vi "DIALOG_Property Selection.vi"(7 "Action":T6, 8 "Error In":errorcluster, 9 "User VI Ref":refnum<vi>, 10 "Affected Items":T4, 11 "Properties for Tree In":T5(array[cluster])=[{"Label"="Divider", "Tag"="0,6,MCListbox (strict),Divider,Divider", "Property Type"=enum."Divider", "Indent"=0, "Can Read?"=FALSE, "Can Write?"=FALSE, "Is Read?"=FALSE, "Is Write?"=FALSE, "Inactive Parent?"=FALSE, "Unwired?"=FALSE}, {"Label"="Class ID", "Tag"="1,1,MCListbox (strict),6327800,Class ID", "Property Type"=enum."Base", "Indent"=0, "Can Read?"=TRUE, "Can Write?"=FALSE, "Is Read?"=FALSE, "Is Write?"=FALSE, "Inactive Parent?"=FALSE, "Unwired?"=FALSE}, {"Label"="Class Name", "Tag"="2,1,MCListbox (strict),6327803,Class Name", "Property Type"=enum."Base", "Indent"=0, "Can Read?"=TRUE, "Can Write?"=FALSE, "Is Read?"=FALSE, "Is Write?"=FALSE, "Inactive Parent?"=FALSE, "Unwired?"=FALSE}, {"Label"="Is On Block Diagram?", "Tag"="3,2,MCListbox (strict),6327805,Is On Block Diagram?", "Property Type"=enum."Scripting", "Indent"=0, "Can Read?"=TRUE, "Can Write?"=FALSE, "Is Read?"=FALSE, "Is Write?"=FALSE, "Inactive Parent?"=FALSE, "Unwired?"=FALSE}, {"Label"="Modified", "Tag"="4,3,MCListbox (strict),6327804,Modified", "Property Type"=enum."Private", "Indent"=0, "Can Read?"=TRUE, "Can Write?"=FALSE, "Is Read?"=FALSE, "Is Write?"=FALSE, "Inactive Parent?"=FALSE, "Unwired?"=FALSE}, {"Label"="Owner", "Tag"="5,1,MCListbox (strict),6327806,Owner", "Property Type"=enum."Base", "Indent"=0, "Can Read?"=TRUE, "Can Write?"=FALSE, "Is Read?"=FALSE, "Is Write?"=FALSE, "Inactive Parent?"=FALSE, "Unwired?"=FALSE}, {"Label"="Owning VI", "Tag"="6,1,MCListbox (strict),6327802,Owning VI", "Property Type"=enum."Base", "Indent"=0, "Can Read?"=TRUE, "Can Write?"=FALSE, "Is Read?"=FALSE, "Is Write?"=FALSE, "Inactive Parent?"=FALSE, "Unwired?"=FALSE}, {"Label"="Divider", "Tag"="7,6,MCListbox (strict),Divider,Divider", "Property Type"=enum."Divider", "Indent"=0, "Can Read?"=FALSE, "Can Write?"=FALSE, "Is Read?"=FALSE, "Is Write?"=FALSE, "Inactive Parent?"=FALSE, "Unwired?"=FALSE}, {"Label"="Basic Object Flags", "Tag"="8,3,MCListbox (strict),632a80c,Basic Object Flags", "Property Type"=enum."Private", "Indent"=0, "Can Read?"=TRUE, "Can Write?"=TRUE, "Is Read?"=FALSE, "Is Write?"=FALSE, "Inactive Parent?"=FALSE, "Unwired?"=FALSE}, {"Label"="Bounds", "Tag"="9,1,MCListbox (strict),632a803,Bounds", "Property Type"=enum."Base", "Indent"=0, "Can Read?"=TRUE, "Can Write?"=FALSE, "Is Read?"=FALSE, "Is Write?"=FALSE, "Inactive Parent?"=FALSE, "Unwired?"=FALSE}, {"Label"="Area Height", "Tag"="10,1,MCListbox (strict),632a805,Bounds:Area Height", "Property Type"=enum."Base", "Indent"=1, "Can Read?"=TRUE, "Can Write?"=FALSE, "Is Read?"=FALSE, "Is Write?"=FALSE, "Inactive Parent?"=FALSE, "Unwired?"=FALSE}, {"Label"="Area Width", "Tag"="11,1,MCListbox (strict),632a804,Bounds:Area Width", "Property Type"=enum."Base", "Indent"=1, "Can Read?"=TRUE, "Can Write?"=FALSE, "Is Read?"=FALSE, "Is Write?"=FALSE, "Inactive Parent?"=FALSE, "Unwired?"=FALSE}, {"Label"="Dependencies", "Tag"="12,2,MCListbox (strict),632a817,Dependencies", "Property Type"=enum."None", "Indent"=0, "Can Read?"=FALSE, "Can Write?"=FALSE, "Is Read?"=FALSE, "Is Write?"=FALSE, "Inactive Parent?"=TRUE, "Unwired?"=FALSE}, {"Label"="Found Dependency Names", "Tag"="13,2,MCListbox (strict),632a817,Dependencies:Found Dependency Names", "Property Type"=enum."Scripting", "Indent"=1, "Can Read?"=TRUE, "Can Write?"=FALSE, "Is Read?"=FALSE, "Is Write?"=FALSE, "Inactive Parent?"=FALSE, "Unwired?"=FALSE}, {"Label"="Found Dependency Paths", "Tag"="14,2,MCListbox (strict),632a816,Dependencies:Found Dependency Paths", "Property Type"=enum."Scripting", "Indent"=1, "Can Read?"=TRUE, "Can Write?"=FALSE, "Is Read?"=FALSE, "Is Write?"=FALSE, "Inactive Parent?"=FALSE, "Unwired?"=FALSE}, {"Label"="Missing Dependency Names", "Tag"="15,2,MCListbox (strict),632a815,Dependencies:Missing Dependency Names", "Property Type"=enum."Scripting", "Indent"=1, "Can Read?"=TRUE, "Can Write?"=FALSE, "Is Read?"=FALSE, "Is Write?"=FALSE, "Inactive Parent?"=FALSE, "Unwired?"=FALSE}, {"Label"="Missing Dependency Paths", "Tag"="16,2,MCListbox (strict),632a814,Dependencies:Missing Dependency Paths", "Property Type"=enum."Scripting", "Indent"=1, "Can Read?"=TRUE, "Can Write?"=FALSE, "Is Read?"=FALSE, "Is Write?"=FALSE, "Inactive Parent?"=FALSE, "Unwired?"=FALSE}, {"Label"="Group Member Refs[]", "Tag"="17,3,MCListbox (strict),632a808,Group Member Refs[]", "Property Type"=enum."Private", "Indent"=0, "Can Read?"=TRUE, "Can Write?"=FALSE, "Is Read?"=FALSE, "Is Write?"=FALSE, "Inactive Parent?"=FALSE, "Unwired?"=FALSE}, {"Label"="Grouped", "Tag"="18,3,MCListbox (strict),632a806,Grouped", "Property Type"=enum."Private", "Indent"=0, "Can Read?"=TRUE, "Can Write?"=FALSE, "Is Read?"=FALSE, "Is Write?"=FALSE, "Inactive Parent?"=FALSE, "Unwired?"=FALSE}, {"Label"="Is Wizard Locked", "Tag"="19,3,MCListbox (strict),632a80d,Is Wizard Locked", "Property Type"=enum."Private", "Indent"=0, "Can Read?"=TRUE, "Can Write?"=FALSE, "Is Read?"=FALSE, "Is Write?"=FALSE, "Inactive Parent?"=FALSE, "Unwired?"=FALSE}, {"Label"="Locked", "Tag"="20,3,MCListbox (strict),632a807,Locked", "Property Type"=enum."Private", "Indent"=0, "Can Read?"=TRUE, "Can Write?"=FALSE, "Is Read?"=FALSE, "Is Write?"=FALSE, "Inactive Parent?"=FALSE, "Unwired?"=FALSE}, {"Label"="Master Bounds Rect", "Tag"="21,2,MCListbox (strict),632a80b,Master Bounds Rect", "Property Type"=enum."Scripting", "Indent"=0, "Can Read?"=TRUE, "Can Write?"=FALSE, "Is Read?"=FALSE, "Is Write?"=FALSE, "Inactive Parent?"=FALSE, "Unwired?"=FALSE}, {"Label"="Position", "Tag"="22,1,MCListbox (strict),632a800,Position", "Property Type"=enum."Base", "Indent"=0, "Can Read?"=TRUE, "Can Write?"=TRUE, "Is Read?"=FALSE, "Is Write?"=FALSE, "Inactive Parent?"=FALSE, "Unwired?"=FALSE}, {"Label"="Left", "Tag"="23,1,MCListbox (strict),632a801,Position:Left", "Property Type"=enum."Base", "Indent"=1, "Can Read?"=TRUE, "Can Write?"=TRUE, "Is Read?"=FALSE, "Is Write?"=FALSE, "Inactive Parent?"=FALSE, "Unwired?"=FALSE}, {"Label"="Top", "Tag"="24,1,MCListbox (strict),632a802,Position:Top", "Property Type"=enum."Base", "Indent"=1, "Can Read?"=TRUE, "Can Write?"=TRUE, "Is Read?"=FALSE, "Is Write?"=FALSE, "Inactive Parent?"=FALSE, "Unwired?"=FALSE}, {"Label"="Resize Info", "Tag"="25,3,MCListbox (strict),632a80f,Resize Info", "Property Type"=enum."None", "Indent"=0, "Can Read?"=FALSE, "Can Write?"=FALSE, "Is Read?"=FALSE, "Is Write?"=FALSE, "Inactive Parent?"=TRUE, "Unwired?"=FALSE}, {"Label"="Can Resize Horizontally", "Tag"="26,3,MCListbox (strict),632a80f,Resize Info:Can Resize Horizontally", "Property Type"=enum."Private", "Indent"=1, "Can Read?"=TRUE, "Can Write?"=FALSE, "Is Read?"=FALSE, "Is Write?"=FALSE, "Inactive Parent?"=FALSE, "Unwired?"=FALSE}, {"Label"="Can Resize Vertically", "Tag"="27,3,MCListbox (strict),632a810,Resize Info:Can Resize Vertically", "Property Type"=enum."Private", "Indent"=1, "Can Read?"=TRUE, "Can Write?"=FALSE, "Is Read?"=FALSE, "Is Write?"=FALSE, "Inactive Parent?"=FALSE, "Unwired?"=FALSE}, {"Label"="Include In Resize", "Tag"="28,3,MCListbox (strict),632a812,Resize Info:Include In Resize", "Property Type"=enum."Private", "Indent"=1, "Can Read?"=TRUE, "Can Write?"=FALSE, "Is Read?"=FALSE, "Is Write?"=FALSE, "Inactive Parent?"=FALSE, "Unwired?"=FALSE}, {"Label"="Name in Resize Dialog", "Tag"="29,3,MCListbox (strict),632a811,Resize Info:Name in Resize Dialog", "Property Type"=enum."Private", "Indent"=1, "Can Read?"=TRUE, "Can Write?"=FALSE, "Is Read?"=FALSE, "Is Write?"=FALSE, "Inactive Parent?"=FALSE, "Unwired?"=FALSE}, {"Label"="Selected", "Tag"="30,2,MCListbox (strict),632a809,Selected", "Property Type"=enum."Scripting", "Indent"=0, "Can Read?"=TRUE, "Can Write?"=TRUE, "Is Read?"=FALSE, "Is Write?"=FALSE, "Inactive Parent?"=FALSE, "Unwired?"=FALSE}, {"Label"="Total Bounds Rect", "Tag"="31,2,MCListbox (strict),632a80a,Total Bounds Rect", "Property Type"=enum."Scripting", "Indent"=0, "Can Read?"=TRUE, "Can Write?"=FALSE, "Is Read?"=FALSE, "Is Write?"=FALSE, "Inactive Parent?"=FALSE, "Unwired?"=FALSE}, {"Label"="UID", "Tag"="32,2,MCListbox (strict),632a813,UID", "Property Type"=enum."Scripting", "Indent"=0, "Can Read?"=TRUE, "Can Write?"=FALSE, "Is Read?"=FALSE, "Is Write?"=FALSE, "Inactive Parent?"=FALSE, "Unwired?"=FALSE}, {"Label"="Divider", "Tag"="33,6,MCListbox (strict),Divider,Divider", "Property Type"=enum."Divider", "Indent"=0, "Can Read?"=FALSE, "Can Write?"=FALSE, "Is Read?"=FALSE, "Is Write?"=FALSE, "Inactive Parent?"=FALSE, "Unwired?"=FALSE}, {"Label"="Auto-Update From Typedef", "Tag"="34,2,MCListbox (strict),633201c,Auto-Update From Typedef", "Property Type"=enum."Scripting", "Indent"=0, "Can Read?"=TRUE, "Can Write?"=TRUE, "Is Read?"=FALSE, "Is Write?"=FALSE, "Inactive Parent?"=FALSE, "Unwired?"=FALSE}, {"Label"="Bit Accurate Data Size", "Tag"="35,3,MCListbox (strict),633201d,Bit Accurate Data Size", "Property Type"=enum."Private", "Indent"=0, "Can Read?"=TRUE, "Can Write?"=FALSE, "Is Read?"=FALSE, "Is Write?"=FALSE, "Inactive Parent?"=FALSE, "Unwired?"=FALSE}, {"Label"="Blinking", "Tag"="36,1,MCListbox (strict),6332003,Blinking", "Property Type"=enum."Base", "Indent"=0, "Can Read?"=TRUE, "Can Write?"=TRUE, "Is Read?"=FALSE, "Is Write?"=FALSE, "Inactive Parent?"=FALSE, "Unwired?"=FALSE}, {"Label"="Built-In Mouse Wheel Support", "Tag"="37,1,MCListbox (strict),633203f,Built-In Mouse Wheel Support", "Property Type"=enum."Base", "Indent"=0, "Can Read?"=TRUE, "Can Write?"=TRUE, "Is Read?"=FALSE, "Is Write?"=FALSE, "Inactive Parent?"=FALSE, "Unwired?"=FALSE}, {"Label"="C Type", "Tag"="38,3,MCListbox (strict),6332026,C Type", "Property Type"=enum."Private", "Indent"=0, "Can Read?"=TRUE, "Can Write?"=FALSE, "Is Read?"=FALSE, "Is Write?"=FALSE, "Inactive Parent?"=FALSE, "Unwired?"=FALSE}, {"Label"="Caption", "Tag"="39,1,MCListbox (strict),6332004,Caption", "Property Type"=enum."Base", "Indent"=0, "Can Read?"=TRUE, "Can Write?"=FALSE, "Is Read?"=FALSE, "Is Write?"=FALSE, "Inactive Parent?"=FALSE, "Unwired?"=FALSE}, {"Label"="Class ID", "Tag"="40,1,MCListbox (strict),6332004.6327800,Caption.Class ID", "Property Type"=enum."Base", "Indent"=1, "Can Read?"=TRUE, "Can Write?"=FALSE, "Is Read?"=FALSE, "Is Write?"=FALSE, "Inactive Parent?"=FALSE, "Unwired?"=FALSE}, {"Label"="Class Name", "Tag"="41,1,MCListbox (strict),6332004.6327803,Caption.Class Name", "Property Type"=enum."Base", "Indent"=1, "Can Read?"=TRUE, "Can Write?"=FALSE, "Is Read?"=FALSE, "Is Write?"=FALSE, "Inactive Parent?"=FALSE, "Unwired?"=FALSE}, {"Label"="Is On Block Diagram?", "Tag"="42,2,MCListbox (strict),6332004.6327805,Caption.Is On Block Diagram?", "Property Type"=enum."Scripting", "Indent"=1, "Can Read?"=TRUE, "Can Write?"=FALSE, "Is Read?"=FALSE, "Is Write?"=FALSE, "Inactive Parent?"=FALSE, "Unwired?"=FALSE}, {"Label"="Modified", "Tag"="43,3,MCListbox (strict),6332004.6327804,Caption.Modified", "Property Type"=enum."Private", "Indent"=1, "Can Read?"=TRUE, "Can Write?"=FALSE, "Is Read?"=FALSE, "Is Write?"=FALSE, "Inactive Parent?"=FALSE, "Unwired?"=FALSE}, {"Label"="Owner", "Tag"="44,1,MCListbox (strict),6332004.6327806,Caption.Owner", "Property Type"=enum."Base", "Indent"=1, "Can Read?"=TRUE, "Can Write?"=FALSE, "Is Read?"=FALSE, "Is Write?"=FALSE, "Inactive Parent?"=FALSE, "Unwired?"=FALSE}, {"Label"="Owning VI", "Tag"="45,1,MCListbox (strict),6332004.6327802,Caption.Owning VI", "Property Type"=enum."Base", "Indent"=1, "Can Read?"=TRUE, "Can Write?"=FALSE, "Is Read?"=FALSE, "Is Write?"=FALSE, "Inactive Parent?"=FALSE, "Unwired?"=FALSE}, {"Label"="Basic Object Flags", "Tag"="46,3,MCListbox (strict),6332004.632a80c,Caption.Basic Object Flags", "Property Type"=enum."Private", "Indent"=1, "Can Read?"=TRUE, "Can Write?"=TRUE, "Is Read?"=FALSE, "Is Write?"=FALSE, "Inactive Parent?"=FALSE, "Unwired?"=FALSE}, {"Label"="Bounds", "Tag"="47,1,MCListbox (strict),6332004.632a803,Caption.Bounds", "Property Type"=enum."Base", "Indent"=1, "Can Read?"=TRUE, "Can Write?"=FALSE, "Is Read?"=FALSE, "Is Write?"=FALSE, "Inactive Parent?"=FALSE, "Unwired?"=FALSE}, {"Label"="Area Height", "Tag"="48,1,MCListbox (strict),6332004.632a805,Caption.Bounds:Area Height", "Property Type"=enum."Base", "Indent"=2, "Can Read?"=TRUE, "Can Write?"=FALSE, "Is Read?"=FALSE, "Is Write?"=FALSE, "Inactive Parent?"=FALSE, "Unwired?"=FALSE}, {"Label"="Area Width", "Tag"="49,1,MCListbox (strict),6332004.632a804,Caption.Bounds:Area Width", "Property Type"=enum."Base", "Indent"=2, "Can Read?"=TRUE, "Can Write?"=FALSE, "Is Read?"=FALSE, "Is Write?"=FALSE, "Inactive Parent?"=FALSE, "Unwired?"=FALSE}, {"Label"="Dependencies", "Tag"="50,2,MCListbox (strict),6332004.632a817,Caption.Dependencies", "Property Type"=enum."None", "Indent"=1, "Can Read?"=FALSE, "Can Write?"=FALSE, "Is Read?"=FALSE, "Is Write?"=FALSE, "Inactive Parent?"=TRUE, "Unwired?"=FALSE}, {"Label"="Found Dependency Names", "Tag"="51,2,MCListbox (strict),6332004.632a817,Caption.Dependencies:Found Dependency Names", "Property Type"=enum."Scripting", "Indent"=2, "Can Read?"=TRUE, "Can Write?"=FALSE, "Is Read?"=FALSE, "Is Write?"=FALSE, "Inactive Parent?"=FALSE, "Unwired?"=FALSE}, {"Label"="Found Dependency Paths", "Tag"="52,2,MCListbox (strict),6332004.632a816,Caption.Dependencies:Found Dependency Paths", "Property Type"=enum."Scripting", "Indent"=2, "Can Read?"=TRUE, "Can Write?"=FALSE, "Is Read?"=FALSE, "Is Write?"=FALSE, "Inactive Parent?"=FALSE, "Unwired?"=FALSE}, {"Label"="Missing Dependency Names", "Tag"="53,2,MCListbox (strict),6332004.632a815,Caption.Dependencies:Missing Dependency Names", "Property Type"=enum."Scripting", "Indent"=2, "Can Read?"=TRUE, "Can Write?"=FALSE, "Is Read?"=FALSE, "Is Write?"=FALSE, "Inactive Parent?"=FALSE, "Unwired?"=FALSE}, {"Label"="Missing Dependency Paths", "Tag"="54,2,MCListbox (strict),6332004.632a814,Caption.Dependencies:Missing Dependency Paths", "Property Type"=enum."Scripting", "Indent"=2, "Can Read?"=TRUE, "Can Write?"=FALSE, "Is Read?"=FALSE, "Is Write?"=FALSE, "Inactive Parent?"=FALSE, "Unwired?"=FALSE}, {"Label"="Group Member Refs[]", "Tag"="55,3,MCListbox (strict),6332004.632a808,Caption.Group Member Refs[]", "Property Type"=enum."Private", "Indent"=1, "Can Read?"=TRUE, "Can Write?"=FALSE, "Is Read?"=FALSE, "Is Write?"=FALSE, "Inactive Parent?"=FALSE, "Unwired?"=FALSE}, {"Label"="Grouped", "Tag"="56,3,MCListbox (strict),6332004.632a806,Caption.Grouped", "Property Type"=enum."Private", "Indent"=1, "Can Read?"=TRUE, "Can Write?"=FALSE, "Is Read?"=FALSE, "Is Write?"=FALSE, "Inactive Parent?"=FALSE, "Unwired?"=FALSE}, {"Label"="Is Wizard Locked", "Tag"="57,3,MCListbox (strict),6332004.632a80d,Caption.Is Wizard Locked", "Property Type"=enum."Private", "Indent"=1, "Can Read?"=TRUE, "Can Write?"=FALSE, "Is Read?"=FALSE, "Is Write?"=FALSE, "Inactive Parent?"=FALSE, "Unwired?"=FALSE}, {"Label"="Locked", "Tag"="58,3,MCListbox (strict),6332004.632a807,Caption.Locked", "Property Type"=enum."Private", "Indent"=1, "Can Read?"=TRUE, "Can Write?"=FALSE, "Is Read?"=FALSE, "Is Write?"=FALSE, "Inactive Parent?"=FALSE, "Unwired?"=FALSE}, {"Label"="Master Bounds Rect", "Tag"="59,2,MCListbox (strict),6332004.632a80b,Caption.Master Bounds Rect", "Property Type"=enum."Scripting", "Indent"=1, "Can Read?"=TRUE, "Can Write?"=FALSE, "Is Read?"=FALSE, "Is Write?"=FALSE, "Inactive Parent?"=FALSE, "Unwired?"=FALSE}, {"Label"="Position", "Tag"="60,1,MCListbox (strict),6332004.632a800,Caption.Position", "Property Type"=enum."Base", "Indent"=1, "Can Read?"=TRUE, "Can Write?"=TRUE, "Is Read?"=FALSE, "Is Write?"=FALSE, "Inactive Parent?"=FALSE, "Unwired?"=FALSE}, {"Label"="Left", "Tag"="61,1,MCListbox (strict),6332004.632a801,Caption.Position:Left", "Property Type"=enum."Base", "Indent"=2, "Can Read?"=TRUE, "Can Write?"=TRUE, "Is Read?"=FALSE, "Is Write?"=FALSE, "Inactive Parent?"=FALSE, "Unwired?"=FALSE}, {"Label"="Top", "Tag"="62,1,MCListbox (strict),6332004.632a802,Caption.Position:Top", "Property Type"=enum."Base", "Indent"=2, "Can Read?"=TRUE, "Can Write?"=TRUE, "Is Read?"=FALSE, "Is Write?"=FALSE, "Inactive Parent?"=FALSE, "Unwired?"=FALSE}, {"Label"="Resize Info", "Tag"="63,3,MCListbox (strict),6332004.632a80f,Caption.Resize Info", "Property Type"=enum."None", "Indent"=1, "Can Read?"=FALSE, "Can Write?"=FALSE, "Is Read?"=FALSE, "Is Write?"=FALSE, "Inactive Parent?"=TRUE, "Unwired?"=FALSE}, {"Label"="Can Resize Horizontally", "Tag"="64,3,MCListbox (strict),6332004.632a80f,Caption.Resize Info:Can Resize Horizontally", "Property Type"=enum."Private", "Indent"=2, "Can Read?"=TRUE, "Can Write?"=FALSE, "Is Read?"=FALSE, "Is Write?"=FALSE, "Inactive Parent?"=FALSE, "Unwired?"=FALSE}, {"Label"="Can Resize Vertically", "Tag"="65,3,MCListbox (strict),6332004.632a810,Caption.Resize Info:Can Resize Vertically", "Property Type"=enum."Private", "Indent"=2, "Can Read?"=TRUE, "Can Write?"=FALSE, "Is Read?"=FALSE, "Is Write?"=FALSE, "Inactive Parent?"=FALSE, "Unwired?"=FALSE}, {"Label"="Include In Resize", "Tag"="66,3,MCListbox (strict),6332004.632a812,Caption.Resize Info:Include In Resize", "Property Type"=enum."Private", "Indent"=2, "Can Read?"=TRUE, "Can Write?"=FALSE, "Is Read?"=FALSE, "Is Write?"=FALSE, "Inactive Parent?"=FALSE, "Unwired?"=FALSE}, {"Label"="Name in Resize Dialog", "Tag"="67,3,MCListbox (strict),6332004.632a811,Caption.Resize Info:Name in Resize Dialog", "Property Type"=enum."Private", "Indent"=2, "Can Read?"=TRUE, "Can Write?"=FALSE, "Is Read?"=FALSE, "Is Write?"=FALSE, "Inactive Parent?"=FALSE, "Unwired?"=FALSE}, {"Label"="Selected", "Tag"="68,2,MCListbox (strict),6332004.632a809,Caption.Selected", "Property Type"=enum."Scripting", "Indent"=1, "Can Read?"=TRUE, "Can Write?"=TRUE, "Is Read?"=FALSE, "Is Write?"=FALSE, "Inactive Parent?"=FALSE, "Unwired?"=FALSE}, {"Label"="Total Bounds Rect", "Tag"="69,2,MCListbox (strict),6332004.632a80a,Caption.Total Bounds Rect", "Property Type"=enum."Scripting", "Indent"=1, "Can Read?"=TRUE, "Can Write?"=FALSE, "Is Read?"=FALSE, "Is Write?"=FALSE, "Inactive Parent?"=FALSE, "Unwired?"=FALSE}, {"Label"="UID", "Tag"="70,2,MCListbox (strict),6332004.632a813,Caption.UID", "Property Type"=enum."Scripting", "Indent"=1, "Can Read?"=TRUE, "Can Write?"=FALSE, "Is Read?"=FALSE, "Is Write?"=FALSE, "Inactive Parent?"=FALSE, "Unwired?"=FALSE}, {"Label"="Colors", "Tag"="71,1,MCListbox (strict),6332004.632cc03,Caption.Colors", "Property Type"=enum."Base", "Indent"=1, "Can Read?"=TRUE, "Can Write?"=TRUE, "Is Read?"=FALSE, "Is Write?"=FALSE, "Inactive Parent?"=FALSE, "Unwired?"=FALSE}, {"Label"="BG Color", "Tag"="72,1,MCListbox (strict),6332004.632cc05,Caption.Colors:BG Color", "Property Type"=enum."Base", "Indent"=2, "Can Read?"=TRUE, "Can Write?"=TRUE, "Is Read?"=FALSE, "Is Write?"=FALSE, "Inactive Parent?"=FALSE, "Unwired?"=FALSE}, {"Label"="FG Color", "Tag"="73,1,MCListbox (strict),6332004.632cc04,Caption.Colors:FG Color", "Property Type"=enum."Base", "Indent"=2, "Can Read?"=TRUE, "Can Write?"=TRUE, "Is Read?"=FALSE, "Is Write?"=FALSE, "Inactive Parent?"=FALSE, "Unwired?"=FALSE}, {"Label"="Owning Pane", "Tag"="74,1,MCListbox (strict),6332004.632cc07,Caption.Owning Pane", "Property Type"=enum."Base", "Indent"=1, "Can Read?"=TRUE, "Can Write?"=FALSE, "Is Read?"=FALSE, "Is Write?"=FALSE, "Inactive Parent?"=FALSE, "Unwired?"=FALSE}, {"Label"="Size", "Tag"="75,1,MCListbox (strict),6332004.632cc00,Caption.Size", "Property Type"=enum."Base", "Indent"=1, "Can Read?"=TRUE, "Can Write?"=TRUE, "Is Read?"=FALSE, "Is Write?"=FALSE, "Inactive Parent?"=FALSE, "Unwired?"=FALSE}, {"Label"="Height", "Tag"="76,1,MCListbox (strict),6332004.632cc02,Caption.Size:Height", "Property Type"=enum."Base", "Indent"=2, "Can Read?"=TRUE, "Can Write?"=TRUE, "Is Read?"=FALSE, "Is Write?"=FALSE, "Inactive Parent?"=FALSE, "Unwired?"=FALSE}, {"Label"="Width", "Tag"="77,1,MCListbox (strict),6332004.632cc01,Caption.Size:Width", "Property Type"=enum."Base", "Indent"=2, "Can Read?"=TRUE, "Can Write?"=TRUE, "Is Read?"=FALSE, "Is Write?"=FALSE, "Inactive Parent?"=FALSE, "Unwired?"=FALSE}, {"Label"="Visible", "Tag"="78,1,MCListbox (strict),6332004.632cc06,Caption.Visible", "Property Type"=enum."Base", "Indent"=1, "Can Read?"=TRUE, "Can Write?"=TRUE, "Is Read?"=FALSE, "Is Write?"=FALSE, "Inactive Parent?"=FALSE, "Unwired?"=FALSE}, {"Label"="Attached Object", "Tag"="79,1,MCListbox (strict),6332004.632d819,Caption.Attached Object", "Property Type"=enum."Base", "Indent"=1, "Can Read?"=TRUE, "Can Write?"=TRUE, "Is Read?"=FALSE, "Is Write?"=FALSE, "Inactive Parent?"=FALSE, "Unwired?"=FALSE}, {"Label"="Document Bounds", "Tag"="80,2,MCListbox (strict),6332004.632d812,Caption.Document Bounds", "Property Type"=enum."Scripting", "Indent"=1, "Can Read?"=TRUE, "Can Write?"=FALSE, "Is Read?"=FALSE, "Is Write?"=FALSE, "Inactive Parent?"=FALSE, "Unwired?"=FALSE}, {"Label"="Height", "Tag"="81,2,MCListbox (strict),6332004.632d814,Caption.Document Bounds:Height", "Property Type"=enum."Scripting", "Indent"=2, "Can Read?"=TRUE, "Can Write?"=FALSE, "Is Read?"=FALSE, "Is Write?"=FALSE, "Inactive Parent?"=FALSE, "Unwired?"=FALSE}, {"Label"="Width", "Tag"="82,2,MCListbox (strict),6332004.632d813,Caption.Document Bounds:Width", "Property Type"=enum."Scripting", "Indent"=2, "Can Read?"=TRUE, "Can Write?"=FALSE, "Is Read?"=FALSE, "Is Write?"=FALSE, "Inactive Parent?"=FALSE, "Unwired?"=FALSE}, {"Label"="Enable Hyperlinks", "Tag"="83,1,MCListbox (strict),6332004.632d81a,Caption.Enable Hyperlinks", "Property Type"=enum."Base", "Indent"=1, "Can Read?"=TRUE, "Can Write?"=TRUE, "Is Read?"=FALSE, "Is Write?"=FALSE, "Inactive Parent?"=FALSE, "Unwired?"=FALSE}, {"Label"="Font", "Tag"="84,1,MCListbox (strict),6332004.632d801,Caption.Font", "Property Type"=enum."Base", "Indent"=1, "Can Read?"=TRUE, "Can Write?"=TRUE, "Is Read?"=FALSE, "Is Write?"=FALSE, "Inactive Parent?"=FALSE, "Unwired?"=FALSE}, {"Label"="Bold", "Tag"="85,1,MCListbox (strict),6332004.632d809,Caption.Font:Bold", "Property Type"=enum."Base", "Indent"=2, "Can Read?"=TRUE, "Can Write?"=TRUE, "Is Read?"=FALSE, "Is Write?"=FALSE, "Inactive Parent?"=FALSE, "Unwired?"=FALSE}, {"Label"="Color", "Tag"="86,1,MCListbox (strict),6332004.632d80d,Caption.Font:Color", "Property Type"=enum."Base", "Indent"=2, "Can Read?"=TRUE, "Can Write?"=TRUE, "Is Read?"=FALSE, "Is Write?"=FALSE, "Inactive Parent?"=FALSE, "Unwired?"=FALSE}, {"Label"="Italic", "Tag"="87,1,MCListbox (strict),6332004.632d80a,Caption.Font:Italic", "Property Type"=enum."Base", "Indent"=2, "Can Read?"=TRUE, "Can Write?"=TRUE, "Is Read?"=FALSE, "Is Write?"=FALSE, "Inactive Parent?"=FALSE, "Unwired?"=FALSE}, {"Label"="Name", "Tag"="88,1,MCListbox (strict),6332004.632d807,Caption.Font:Name", "Property Type"=enum."Base", "Indent"=2, "Can Read?"=TRUE, "Can Write?"=TRUE, "Is Read?"=FALSE, "Is Write?"=FALSE, "Inactive Parent?"=FALSE, "Unwired?"=FALSE}, {"Label"="Size", "Tag"="89,1,MCListbox (strict),6332004.632d808,Caption.Font:Size", "Property Type"=enum."Base", "Indent"=2, "Can Read?"=TRUE, "Can Write?"=TRUE, "Is Read?"=FALSE, "Is Write?"=FALSE, "Inactive Parent?"=FALSE, "Unwired?"=FALSE}, {"Label"="Strikeout", "Tag"="90,1,MCListbox (strict),6332004.632d80c,Caption.Font:Strikeout", "Property Type"=enum."Base", "Indent"=2, "Can Read?"=TRUE, "Can Write?"=TRUE, "Is Read?"=FALSE, "Is Write?"=FALSE, "Inactive Parent?"=FALSE, "Unwired?"=FALSE}, {"Label"="Underline", "Tag"="91,1,MCListbox (strict),6332004.632d80b,Caption.Font:Underline", "Property Type"=enum."Base", "Indent"=2, "Can Read?"=TRUE, "Can Write?"=TRUE, "Is Read?"=FALSE, "Is Write?"=FALSE, "Inactive Parent?"=FALSE, "Unwired?"=FALSE}, {"Label"="FontType", "Tag"="92,3,MCListbox (strict),6332004.632d818,Caption.FontType", "Property Type"=enum."Private", "Indent"=1, "Can Read?"=FALSE, "Can Write?"=TRUE, "Is Read?"=FALSE, "Is Write?"=FALSE, "Inactive Parent?"=FALSE, "Unwired?"=FALSE}, {"Label"="Interpret As Unicode", "Tag"="93,3,MCListbox (strict),6332004.632d811,Caption.Interpret As Unicode", "Property Type"=enum."Private", "Indent"=1, "Can Read?"=TRUE, "Can Write?"=TRUE, "Is Read?"=FALSE, "Is Write?"=FALSE, "Inactive Parent?"=FALSE, "Unwired?"=FALSE}, {"Label"="Justification", "Tag"="94,1,MCListbox (strict),6332004.632d815,Caption.Justification", "Property Type"=enum."Base", "Indent"=1, "Can Read?"=TRUE, "Can Write?"=TRUE, "Is Read?"=FALSE, "Is Write?"=FALSE, "Inactive Parent?"=FALSE, "Unwired?"=FALSE}, {"Label"="Lock", "Tag"="95,1,MCListbox (strict),6332004.632d817,Caption.Lock", "Property Type"=enum."Base", "Indent"=1, "Can Read?"=TRUE, "Can Write?"=TRUE, "Is Read?"=FALSE, "Is Write?"=FALSE, "Inactive Parent?"=FALSE, "Unwired?"=FALSE}, {"Label"="Scroll Position", "Tag"="96,1,MCListbox (strict),6332004.632d805,Caption.Scroll Position", "Property Type"=enum."Base", "Indent"=1, "Can Read?"=TRUE, "Can Write?"=TRUE, "Is Read?"=FALSE, "Is Write?"=FALSE, "Inactive Parent?"=FALSE, "Unwired?"=FALSE}, {"Label"="Selection", "Tag"="97,1,MCListbox (strict),6332004.632d802,Caption.Selection", "Property Type"=enum."Base", "Indent"=1, "Can Read?"=TRUE, "Can Write?"=TRUE, "Is Read?"=FALSE, "Is Write?"=FALSE, "Inactive Parent?"=FALSE, "Unwired?"=FALSE}, {"Label"="End", "Tag"="98,1,MCListbox (strict),6332004.632d804,Caption.Selection:End", "Property Type"=enum."Base", "Indent"=2, "Can Read?"=TRUE, "Can Write?"=TRUE, "Is Read?"=FALSE, "Is Write?"=FALSE, "Inactive Parent?"=FALSE, "Unwired?"=FALSE}, {"Label"="Start", "Tag"="99,1,MCListbox (strict),6332004.632d803,Caption.Selection:Start", "Property Type"=enum."Base", "Indent"=2, "Can Read?"=TRUE, "Can Write?"=TRUE, "Is Read?"=FALSE, "Is Write?"=FALSE, "Inactive Parent?"=FALSE, "Unwired?"=FALSE}, {"Label"="Size to Text?", "Tag"="100,1,MCListbox (strict),6332004.632d806,Caption.Size to Text?", "Property Type"=enum."Base", "Indent"=1, "Can Read?"=TRUE, "Can Write?"=TRUE, "Is Read?"=FALSE, "Is Write?"=FALSE, "Inactive Parent?"=FALSE, "Unwired?"=FALSE}, {"Label"="Text", "Tag"="101,1,MCListbox (strict),6332004.632d800,Caption.Text", "Property Type"=enum."Base", "Indent"=1, "Can Read?"=TRUE, "Can Write?"=TRUE, "Is Read?"=FALSE, "Is Write?"=FALSE, "Inactive Parent?"=FALSE, "Unwired?"=FALSE}, {"Label"="Text Colors", "Tag"="102,1,MCListbox (strict),6332004.632d80e,Caption.Text Colors", "Property Type"=enum."Base", "Indent"=1, "Can Read?"=TRUE, "Can Write?"=TRUE, "Is Read?"=FALSE, "Is Write?"=FALSE, "Inactive Parent?"=FALSE, "Unwired?"=FALSE}, {"Label"="BG Color", "Tag"="103,1,MCListbox (strict),6332004.632d810,Caption.Text Colors:BG Color", "Property Type"=enum."Base", "Indent"=2, "Can Read?"=TRUE, "Can Write?"=TRUE, "Is Read?"=FALSE, "Is Write?"=FALSE, "Inactive Parent?"=FALSE, "Unwired?"=FALSE}, {"Label"="Text Color", "Tag"="104,1,MCListbox (strict),6332004.632d80f,Caption.Text Colors:Text Color", "Property Type"=enum."Base", "Indent"=2, "Can Read?"=TRUE, "Can Write?"=TRUE, "Is Read?"=FALSE, "Is Write?"=FALSE, "Inactive Parent?"=FALSE, "Unwired?"=FALSE}, {"Label"="Text Overflow", "Tag"="105,1,MCListbox (strict),6332004.632d81b,Caption.Text Overflow", "Property Type"=enum."Base", "Indent"=1, "Can Read?"=TRUE, "Can Write?"=TRUE, "Is Read?"=FALSE, "Is Write?"=FALSE, "Inactive Parent?"=FALSE, "Unwired?"=FALSE}, {"Label"="Vertical Arrangement", "Tag"="106,1,MCListbox (strict),6332004.632d816,Caption.Vertical Arrangement", "Property Type"=enum."Base", "Indent"=1, "Can Read?"=TRUE, "Can Write?"=TRUE, "Is Read?"=FALSE, "Is Write?"=FALSE, "Inactive Parent?"=FALSE, "Unwired?"=FALSE}, {"Label"="Control Index", "Tag"="107,1,MCListbox (strict),6332040,Control Index", "Property Type"=enum."Base", "Indent"=0, "Can Read?"=TRUE, "Can Write?"=FALSE, "Is Read?"=FALSE, "Is Write?"=FALSE, "Inactive Parent?"=FALSE, "Unwired?"=FALSE}, {"Label"="Control Reference Nodes[]", "Tag"="108,2,MCListbox (strict),6332009,Control Reference Nodes[]", "Property Type"=enum."Scripting", "Indent"=0, "Can Read?"=TRUE, "Can Write?"=FALSE, "Is Read?"=FALSE, "Is Write?"=FALSE, "Inactive Parent?"=FALSE, "Unwired?"=FALSE}, {"Label"="Data Binding", "Tag"="109,1,MCListbox (strict),633202d,Data Binding", "Property Type"=enum."None", "Indent"=0, "Can Read?"=FALSE, "Can Write?"=FALSE, "Is Read?"=FALSE, "Is Write?"=FALSE, "Inactive Parent?"=TRUE, "Unwired?"=FALSE}, {"Label"="Binding Type", "Tag"="110,1,MCListbox (strict),633202d,Data Binding:Binding Type", "Property Type"=enum."Base", "Indent"=1, "Can Read?"=TRUE, "Can Write?"=FALSE, "Is Read?"=FALSE, "Is Write?"=FALSE, "Inactive Parent?"=FALSE, "Unwired?"=FALSE}, {"Label"="Blink On Alarm", "Tag"="111,3,MCListbox (strict),633202e,Data Binding:Blink On Alarm", "Property Type"=enum."Private", "Indent"=1, "Can Read?"=TRUE, "Can Write?"=TRUE, "Is Read?"=FALSE, "Is Write?"=FALSE, "Inactive Parent?"=FALSE, "Unwired?"=FALSE}, {"Label"="LED Visible", "Tag"="112,1,MCListbox (strict),633202b,Data Binding:LED Visible", "Property Type"=enum."Base", "Indent"=1, "Can Read?"=TRUE, "Can Write?"=TRUE, "Is Read?"=FALSE, "Is Write?"=FALSE, "Inactive Parent?"=FALSE, "Unwired?"=FALSE}, {"Label"="Mode", "Tag"="113,1,MCListbox (strict),6332029,Data Binding:Mode", "Property Type"=enum."Base", "Indent"=1, "Can Read?"=TRUE, "Can Write?"=TRUE, "Is Read?"=FALSE, "Is Write?"=FALSE, "Inactive Parent?"=FALSE, "Unwired?"=FALSE}, {"Label"="Path", "Tag"="114,1,MCListbox (strict),6332028,Data Binding:Path", "Property Type"=enum."Base", "Indent"=1, "Can Read?"=TRUE, "Can Write?"=TRUE, "Is Read?"=FALSE, "Is Write?"=FALSE, "Inactive Parent?"=FALSE, "Unwired?"=FALSE}, {"Label"="Persist ID", "Tag"="115,3,MCListbox (strict),633202c,Data Binding:Persist ID", "Property Type"=enum."Private", "Indent"=1, "Can Read?"=TRUE, "Can Write?"=FALSE, "Is Read?"=FALSE, "Is Write?"=FALSE, "Inactive Parent?"=FALSE, "Unwired?"=FALSE}, {"Label"="Status", "Tag"="116,1,MCListbox (strict),633202a,Data Binding:Status", "Property Type"=enum."Base", "Indent"=1, "Can Read?"=TRUE, "Can Write?"=FALSE, "Is Read?"=FALSE, "Is Write?"=FALSE, "Inactive Parent?"=FALSE, "Unwired?"=FALSE}, {"Label"="DataSocket", "Tag"="117,1,MCListbox (strict),6332017,DataSocket", "Property Type"=enum."None", "Indent"=0, "Can Read?"=FALSE, "Can Write?"=FALSE, "Is Read?"=FALSE, "Is Write?"=FALSE, "Inactive Parent?"=TRUE, "Unwired?"=FALSE}, {"Label"="Enabled", "Tag"="118,1,MCListbox (strict),6332017,DataSocket:Enabled", "Property Type"=enum."Base", "Indent"=1, "Can Read?"=TRUE, "Can Write?"=TRUE, "Is Read?"=FALSE, "Is Write?"=FALSE, "Inactive Parent?"=FALSE, "Unwired?"=FALSE}, {"Label"="LED Visible", "Tag"="119,1,MCListbox (strict),633201e,DataSocket:LED Visible", "Property Type"=enum."Base", "Indent"=1, "Can Read?"=TRUE, "Can Write?"=TRUE, "Is Read?"=FALSE, "Is Write?"=FALSE, "Inactive Parent?"=FALSE, "Unwired?"=FALSE}, {"Label"="Mode", "Tag"="120,1,MCListbox (strict),6332016,DataSocket:Mode", "Property Type"=enum."Base", "Indent"=1, "Can Read?"=TRUE, "Can Write?"=TRUE, "Is Read?"=FALSE, "Is Write?"=FALSE, "Inactive Parent?"=FALSE, "Unwired?"=FALSE}, {"Label"="Status", "Tag"="121,1,MCListbox (strict),6332018,DataSocket:Status", "Property Type"=enum."Base", "Indent"=1, "Can Read?"=TRUE, "Can Write?"=FALSE, "Is Read?"=FALSE, "Is Write?"=FALSE, "Inactive Parent?"=FALSE, "Unwired?"=FALSE}, {"Label"="URL", "Tag"="122,1,MCListbox (strict),6332015,DataSocket:URL", "Property Type"=enum."Base", "Indent"=1, "Can Read?"=TRUE, "Can Write?"=TRUE, "Is Read?"=FALSE, "Is Write?"=FALSE, "Inactive Parent?"=FALSE, "Unwired?"=FALSE}, {"Label"="Default Value", "Tag"="123,2,MCListbox (strict),6332013,Default Value", "Property Type"=enum."Scripting", "Indent"=0, "Can Read?"=TRUE, "Can Write?"=TRUE, "Is Read?"=FALSE, "Is Write?"=FALSE, "Inactive Parent?"=FALSE, "Unwired?"=FALSE}, {"Label"="Default Value (Undoable)", "Tag"="124,2,MCListbox (strict),6332043,Default Value (Undoable)", "Property Type"=enum."Scripting", "Indent"=0, "Can Read?"=FALSE, "Can Write?"=TRUE, "Is Read?"=FALSE, "Is Write?"=FALSE, "Inactive Parent?"=FALSE, "Unwired?"=FALSE}, {"Label"="Description", "Tag"="125,1,MCListbox (strict),633200f,Description", "Property Type"=enum."Base", "Indent"=0, "Can Read?"=TRUE, "Can Write?"=TRUE, "Is Read?"=FALSE, "Is Write?"=FALSE, "Inactive Parent?"=FALSE, "Unwired?"=FALSE}, {"Label"="Disabled", "Tag"="126,1,MCListbox (strict),633203d,Disabled", "Property Type"=enum."Base", "Indent"=0, "Can Read?"=TRUE, "Can Write?"=TRUE, "Is Read?"=FALSE, "Is Write?"=FALSE, "Inactive Parent?"=FALSE, "Unwired?"=FALSE}, {"Label"="Focus Key Binding", "Tag"="127,1,MCListbox (strict),6332010,Focus Key Binding", "Property Type"=enum."Base", "Indent"=0, "Can Read?"=TRUE, "Can Write?"=TRUE, "Is Read?"=FALSE, "Is Write?"=FALSE, "Inactive Parent?"=FALSE, "Unwired?"=FALSE}, {"Label"="Genericity", "Tag"="128,3,MCListbox (strict),633203c,Genericity", "Property Type"=enum."Private", "Indent"=0, "Can Read?"=TRUE, "Can Write?"=TRUE, "Is Read?"=FALSE, "Is Write?"=FALSE, "Inactive Parent?"=FALSE, "Unwired?"=FALSE}, {"Label"="Grow Info", "Tag"="129,2,MCListbox (strict),633202f,Grow Info", "Property Type"=enum."Scripting", "Indent"=0, "Can Read?"=TRUE, "Can Write?"=FALSE, "Is Read?"=FALSE, "Is Write?"=FALSE, "Inactive Parent?"=FALSE, "Unwired?"=FALSE}, {"Label"="Can Grow Horizontally", "Tag"="130,2,MCListbox (strict),6332030,Grow Info:Can Grow Horizontally", "Property Type"=enum."Scripting", "Indent"=1, "Can Read?"=TRUE, "Can Write?"=FALSE, "Is Read?"=FALSE, "Is Write?"=FALSE, "Inactive Parent?"=FALSE, "Unwired?"=FALSE}, {"Label"="Can Grow Vertically", "Tag"="131,2,MCListbox (strict),6332031,Grow Info:Can Grow Vertically", "Property Type"=enum."Scripting", "Indent"=1, "Can Read?"=TRUE, "Can Write?"=FALSE, "Is Read?"=FALSE, "Is Write?"=FALSE, "Inactive Parent?"=FALSE, "Unwired?"=FALSE}, {"Label"="Max Horizontally", "Tag"="132,2,MCListbox (strict),6332034,Grow Info:Max Horizontally", "Property Type"=enum."Scripting", "Indent"=1, "Can Read?"=TRUE, "Can Write?"=FALSE, "Is Read?"=FALSE, "Is Write?"=FALSE, "Inactive Parent?"=FALSE, "Unwired?"=FALSE}, {"Label"="Max Vertically", "Tag"="133,2,MCListbox (strict),6332035,Grow Info:Max Vertically", "Property Type"=enum."Scripting", "Indent"=1, "Can Read?"=TRUE, "Can Write?"=FALSE, "Is Read?"=FALSE, "Is Write?"=FALSE, "Inactive Parent?"=FALSE, "Unwired?"=FALSE}, {"Label"="Min Horizontally", "Tag"="134,2,MCListbox (strict),6332032,Grow Info:Min Horizontally", "Property Type"=enum."Scripting", "Indent"=1, "Can Read?"=TRUE, "Can Write?"=FALSE, "Is Read?"=FALSE, "Is Write?"=FALSE, "Inactive Parent?"=FALSE, "Unwired?"=FALSE}, {"Label"="Min Vertically", "Tag"="135,2,MCListbox (strict),6332033,Grow Info:Min Vertically", "Property Type"=enum."Scripting", "Indent"=1, "Can Read?"=TRUE, "Can Write?"=FALSE, "Is Read?"=FALSE, "Is Write?"=FALSE, "Inactive Parent?"=FALSE, "Unwired?"=FALSE}, {"Label"="Has Caption", "Tag"="136,2,MCListbox (strict),6332022,Has Caption", "Property Type"=enum."Scripting", "Indent"=0, "Can Read?"=TRUE, "Can Write?"=FALSE, "Is Read?"=FALSE, "Is Write?"=FALSE, "Inactive Parent?"=FALSE, "Unwired?"=FALSE}, {"Label"="Indicator", "Tag"="137,1,MCListbox (strict),6332007,Indicator", "Property Type"=enum."Base", "Indent"=0, "Can Read?"=TRUE, "Can Write?"=TRUE, "Is Read?"=FALSE, "Is Write?"=FALSE, "Inactive Parent?"=FALSE, "Unwired?"=FALSE}, {"Label"="Invoke Nodes[]", "Tag"="138,2,MCListbox (strict),633200c,Invoke Nodes[]", "Property Type"=enum."Scripting", "Indent"=0, "Can Read?"=TRUE, "Can Write?"=FALSE, "Is Read?"=FALSE, "Is Write?"=FALSE, "Inactive Parent?"=FALSE, "Unwired?"=FALSE}, {"Label"="Is On Connector Pane", "Tag"="139,2,MCListbox (strict),6332020,Is On Connector Pane", "Property Type"=enum."Scripting", "Indent"=0, "Can Read?"=TRUE, "Can Write?"=FALSE, "Is Read?"=FALSE, "Is Write?"=FALSE, "Inactive Parent?"=FALSE, "Unwired?"=FALSE}, {"Label"="Is Stub?", "Tag"="140,3,MCListbox (strict),633203b,Is Stub?", "Property Type"=enum."Private", "Indent"=0, "Can Read?"=TRUE, "Can Write?"=FALSE, "Is Read?"=FALSE, "Is Write?"=FALSE, "Inactive Parent?"=FALSE, "Unwired?"=FALSE}, {"Label"="Is Typedef?", "Tag"="141,2,MCListbox (strict),633201a,Is Typedef?", "Property Type"=enum."Scripting", "Indent"=0, "Can Read?"=TRUE, "Can Write?"=FALSE, "Is Read?"=FALSE, "Is Write?"=FALSE, "Inactive Parent?"=FALSE, "Unwired?"=FALSE}, {"Label"="Key Focus", "Tag"="142,1,MCListbox (strict),6332002,Key Focus", "Property Type"=enum."Base", "Indent"=0, "Can Read?"=TRUE, "Can Write?"=TRUE, "Is Read?"=FALSE, "Is Write?"=FALSE, "Inactive Parent?"=FALSE, "Unwired?"=FALSE}, {"Label"="Label", "Tag"="143,1,MCListbox (strict),6332005,Label", "Property Type"=enum."Base", "Indent"=0, "Can Read?"=TRUE, "Can Write?"=FALSE, "Is Read?"=FALSE, "Is Write?"=FALSE, "Inactive Parent?"=FALSE, "Unwired?"=FALSE}, {"Label"="Class ID", "Tag"="144,1,MCListbox (strict),6332005.6327800,Label.Class ID", "Property Type"=enum."Base", "Indent"=1, "Can Read?"=TRUE, "Can Write?"=FALSE, "Is Read?"=FALSE, "Is Write?"=FALSE, "Inactive Parent?"=FALSE, "Unwired?"=FALSE}, {"Label"="Class Name", "Tag"="145,1,MCListbox (strict),6332005.6327803,Label.Class Name", "Property Type"=enum."Base", "Indent"=1, "Can Read?"=TRUE, "Can Write?"=FALSE, "Is Read?"=FALSE, "Is Write?"=FALSE, "Inactive Parent?"=FALSE, "Unwired?"=FALSE}, {"Label"="Is On Block Diagram?", "Tag"="146,2,MCListbox (strict),6332005.6327805,Label.Is On Block Diagram?", "Property Type"=enum."Scripting", "Indent"=1, "Can Read?"=TRUE, "Can Write?"=FALSE, "Is Read?"=FALSE, "Is Write?"=FALSE, "Inactive Parent?"=FALSE, "Unwired?"=FALSE}, {"Label"="Modified", "Tag"="147,3,MCListbox (strict),6332005.6327804,Label.Modified", "Property Type"=enum."Private", "Indent"=1, "Can Read?"=TRUE, "Can Write?"=FALSE, "Is Read?"=FALSE, "Is Write?"=FALSE, "Inactive Parent?"=FALSE, "Unwired?"=FALSE}, {"Label"="Owner", "Tag"="148,1,MCListbox (strict),6332005.6327806,Label.Owner", "Property Type"=enum."Base", "Indent"=1, "Can Read?"=TRUE, "Can Write?"=FALSE, "Is Read?"=FALSE, "Is Write?"=FALSE, "Inactive Parent?"=FALSE, "Unwired?"=FALSE}, {"Label"="Owning VI", "Tag"="149,1,MCListbox (strict),6332005.6327802,Label.Owning VI", "Property Type"=enum."Base", "Indent"=1, "Can Read?"=TRUE, "Can Write?"=FALSE, "Is Read?"=FALSE, "Is Write?"=FALSE, "Inactive Parent?"=FALSE, "Unwired?"=FALSE}, {"Label"="Basic Object Flags", "Tag"="150,3,MCListbox (strict),6332005.632a80c,Label.Basic Object Flags", "Property Type"=enum."Private", "Indent"=1, "Can Read?"=TRUE, "Can Write?"=TRUE, "Is Read?"=FALSE, "Is Write?"=FALSE, "Inactive Parent?"=FALSE, "Unwired?"=FALSE}, {"Label"="Bounds", "Tag"="151,1,MCListbox (strict),6332005.632a803,Label.Bounds", "Property Type"=enum."Base", "Indent"=1, "Can Read?"=TRUE, "Can Write?"=FALSE, "Is Read?"=FALSE, "Is Write?"=FALSE, "Inactive Parent?"=FALSE, "Unwired?"=FALSE}, {"Label"="Area Height", "Tag"="152,1,MCListbox (strict),6332005.632a805,Label.Bounds:Area Height", "Property Type"=enum."Base", "Indent"=2, "Can Read?"=TRUE, "Can Write?"=FALSE, "Is Read?"=FALSE, "Is Write?"=FALSE, "Inactive Parent?"=FALSE, "Unwired?"=FALSE}, {"Label"="Area Width", "Tag"="153,1,MCListbox (strict),6332005.632a804,Label.Bounds:Area Width", "Property Type"=enum."Base", "Indent"=2, "Can Read?"=TRUE, "Can Write?"=FALSE, "Is Read?"=FALSE, "Is Write?"=FALSE, "Inactive Parent?"=FALSE, "Unwired?"=FALSE}, {"Label"="Dependencies", "Tag"="154,2,MCListbox (strict),6332005.632a817,Label.Dependencies", "Property Type"=enum."None", "Indent"=1, "Can Read?"=FALSE, "Can Write?"=FALSE, "Is Read?"=FALSE, "Is Write?"=FALSE, "Inactive Parent?"=TRUE, "Unwired?"=FALSE}, {"Label"="Found Dependency Names", "Tag"="155,2,MCListbox (strict),6332005.632a817,Label.Dependencies:Found Dependency Names", "Property Type"=enum."Scripting", "Indent"=2, "Can Read?"=TRUE, "Can Write?"=FALSE, "Is Read?"=FALSE, "Is Write?"=FALSE, "Inactive Parent?"=FALSE, "Unwired?"=FALSE}, {"Label"="Found Dependency Paths", "Tag"="156,2,MCListbox (strict),6332005.632a816,Label.Dependencies:Found Dependency Paths", "Property Type"=enum."Scripting", "Indent"=2, "Can Read?"=TRUE, "Can Write?"=FALSE, "Is Read?"=FALSE, "Is Write?"=FALSE, "Inactive Parent?"=FALSE, "Unwired?"=FALSE}, {"Label"="Missing Dependency Names", "Tag"="157,2,MCListbox (strict),6332005.632a815,Label.Dependencies:Missing Dependency Names", "Property Type"=enum."Scripting", "Indent"=2, "Can Read?"=TRUE, "Can Write?"=FALSE, "Is Read?"=FALSE, "Is Write?"=FALSE, "Inactive Parent?"=FALSE, "Unwired?"=FALSE}, {"Label"="Missing Dependency Paths", "Tag"="158,2,MCListbox (strict),6332005.632a814,Label.Dependencies:Missing Dependency Paths", "Property Type"=enum."Scripting", "Indent"=2, "Can Read?"=TRUE, "Can Write?"=FALSE, "Is Read?"=FALSE, "Is Write?"=FALSE, "Inactive Parent?"=FALSE, "Unwired?"=FALSE}, {"Label"="Group Member Refs[]", "Tag"="159,3,MCListbox (strict),6332005.632a808,Label.Group Member Refs[]", "Property Type"=enum."Private", "Indent"=1, "Can Read?"=TRUE, "Can Write?"=FALSE, "Is Read?"=FALSE, "Is Write?"=FALSE, "Inactive Parent?"=FALSE, "Unwired?"=FALSE}, {"Label"="Grouped", "Tag"="160,3,MCListbox (strict),6332005.632a806,Label.Grouped", "Property Type"=enum."Private", "Indent"=1, "Can Read?"=TRUE, "Can Write?"=FALSE, "Is Read?"=FALSE, "Is Write?"=FALSE, "Inactive Parent?"=FALSE, "Unwired?"=FALSE}, {"Label"="Is Wizard Locked", "Tag"="161,3,MCListbox (strict),6332005.632a80d,Label.Is Wizard Locked", "Property Type"=enum."Private", "Indent"=1, "Can Read?"=TRUE, "Can Write?"=FALSE, "Is Read?"=FALSE, "Is Write?"=FALSE, "Inactive Parent?"=FALSE, "Unwired?"=FALSE}, {"Label"="Locked", "Tag"="162,3,MCListbox (strict),6332005.632a807,Label.Locked", "Property Type"=enum."Private", "Indent"=1, "Can Read?"=TRUE, "Can Write?"=FALSE, "Is Read?"=FALSE, "Is Write?"=FALSE, "Inactive Parent?"=FALSE, "Unwired?"=FALSE}, {"Label"="Master Bounds Rect", "Tag"="163,2,MCListbox (strict),6332005.632a80b,Label.Master Bounds Rect", "Property Type"=enum."Scripting", "Indent"=1, "Can Read?"=TRUE, "Can Write?"=FALSE, "Is Read?"=FALSE, "Is Write?"=FALSE, "Inactive Parent?"=FALSE, "Unwired?"=FALSE}, {"Label"="Position", "Tag"="164,1,MCListbox (strict),6332005.632a800,Label.Position", "Property Type"=enum."Base", "Indent"=1, "Can Read?"=TRUE, "Can Write?"=TRUE, "Is Read?"=FALSE, "Is Write?"=FALSE, "Inactive Parent?"=FALSE, "Unwired?"=FALSE}, {"Label"="Left", "Tag"="165,1,MCListbox (strict),6332005.632a801,Label.Position:Left", "Property Type"=enum."Base", "Indent"=2, "Can Read?"=TRUE, "Can Write?"=TRUE, "Is Read?"=FALSE, "Is Write?"=FALSE, "Inactive Parent?"=FALSE, "Unwired?"=FALSE}, {"Label"="Top", "Tag"="166,1,MCListbox (strict),6332005.632a802,Label.Position:Top", "Property Type"=enum."Base", "Indent"=2, "Can Read?"=TRUE, "Can Write?"=TRUE, "Is Read?"=FALSE, "Is Write?"=FALSE, "Inactive Parent?"=FALSE, "Unwired?"=FALSE}, {"Label"="Resize Info", "Tag"="167,3,MCListbox (strict),6332005.632a80f,Label.Resize Info", "Property Type"=enum."None", "Indent"=1, "Can Read?"=FALSE, "Can Write?"=FALSE, "Is Read?"=FALSE, "Is Write?"=FALSE, "Inactive Parent?"=TRUE, "Unwired?"=FALSE}, {"Label"="Can Resize Horizontally", "Tag"="168,3,MCListbox (strict),6332005.632a80f,Label.Resize Info:Can Resize Horizontally", "Property Type"=enum."Private", "Indent"=2, "Can Read?"=TRUE, "Can Write?"=FALSE, "Is Read?"=FALSE, "Is Write?"=FALSE, "Inactive Parent?"=FALSE, "Unwired?"=FALSE}, {"Label"="Can Resize Vertically", "Tag"="169,3,MCListbox (strict),6332005.632a810,Label.Resize Info:Can Resize Vertically", "Property Type"=enum."Private", "Indent"=2, "Can Read?"=TRUE, "Can Write?"=FALSE, "Is Read?"=FALSE, "Is Write?"=FALSE, "Inactive Parent?"=FALSE, "Unwired?"=FALSE}, {"Label"="Include In Resize", "Tag"="170,3,MCListbox (strict),6332005.632a812,Label.Resize Info:Include In Resize", "Property Type"=enum."Private", "Indent"=2, "Can Read?"=TRUE, "Can Write?"=FALSE, "Is Read?"=FALSE, "Is Write?"=FALSE, "Inactive Parent?"=FALSE, "Unwired?"=FALSE}, {"Label"="Name in Resize Dialog", "Tag"="171,3,MCListbox (strict),6332005.632a811,Label.Resize Info:Name in Resize Dialog", "Property Type"=enum."Private", "Indent"=2, "Can Read?"=TRUE, "Can Write?"=FALSE, "Is Read?"=FALSE, "Is Write?"=FALSE, "Inactive Parent?"=FALSE, "Unwired?"=FALSE}, {"Label"="Selected", "Tag"="172,2,MCListbox (strict),6332005.632a809,Label.Selected", "Property Type"=enum."Scripting", "Indent"=1, "Can Read?"=TRUE, "Can Write?"=TRUE, "Is Read?"=FALSE, "Is Write?"=FALSE, "Inactive Parent?"=FALSE, "Unwired?"=FALSE}, {"Label"="Total Bounds Rect", "Tag"="173,2,MCListbox (strict),6332005.632a80a,Label.Total Bounds Rect", "Property Type"=enum."Scripting", "Indent"=1, "Can Read?"=TRUE, "Can Write?"=FALSE, "Is Read?"=FALSE, "Is Write?"=FALSE, "Inactive Parent?"=FALSE, "Unwired?"=FALSE}, {"Label"="UID", "Tag"="174,2,MCListbox (strict),6332005.632a813,Label.UID", "Property Type"=enum."Scripting", "Indent"=1, "Can Read?"=TRUE, "Can Write?"=FALSE, "Is Read?"=FALSE, "Is Write?"=FALSE, "Inactive Parent?"=FALSE, "Unwired?"=FALSE}, {"Label"="Colors", "Tag"="175,1,MCListbox (strict),6332005.632cc03,Label.Colors", "Property Type"=enum."Base", "Indent"=1, "Can Read?"=TRUE, "Can Write?"=TRUE, "Is Read?"=FALSE, "Is Write?"=FALSE, "Inactive Parent?"=FALSE, "Unwired?"=FALSE}, {"Label"="BG Color", "Tag"="176,1,MCListbox (strict),6332005.632cc05,Label.Colors:BG Color", "Property Type"=enum."Base", "Indent"=2, "Can Read?"=TRUE, "Can Write?"=TRUE, "Is Read?"=FALSE, "Is Write?"=FALSE, "Inactive Parent?"=FALSE, "Unwired?"=FALSE}, {"Label"="FG Color", "Tag"="177,1,MCListbox (strict),6332005.632cc04,Label.Colors:FG Color", "Property Type"=enum."Base", "Indent"=2, "Can Read?"=TRUE, "Can Write?"=TRUE, "Is Read?"=FALSE, "Is Write?"=FALSE, "Inactive Parent?"=FALSE, "Unwired?"=FALSE}, {"Label"="Owning Pane", "Tag"="178,1,MCListbox (strict),6332005.632cc07,Label.Owning Pane", "Property Type"=enum."Base", "Indent"=1, "Can Read?"=TRUE, "Can Write?"=FALSE, "Is Read?"=FALSE, "Is Write?"=FALSE, "Inactive Parent?"=FALSE, "Unwired?"=FALSE}, {"Label"="Size", "Tag"="179,1,MCListbox (strict),6332005.632cc00,Label.Size", "Property Type"=enum."Base", "Indent"=1, "Can Read?"=TRUE, "Can Write?"=TRUE, "Is Read?"=FALSE, "Is Write?"=FALSE, "Inactive Parent?"=FALSE, "Unwired?"=FALSE}, {"Label"="Height", "Tag"="180,1,MCListbox (strict),6332005.632cc02,Label.Size:Height", "Property Type"=enum."Base", "Indent"=2, "Can Read?"=TRUE, "Can Write?"=TRUE, "Is Read?"=FALSE, "Is Write?"=FALSE, "Inactive Parent?"=FALSE, "Unwired?"=FALSE}, {"Label"="Width", "Tag"="181,1,MCListbox (strict),6332005.632cc01,Label.Size:Width", "Property Type"=enum."Base", "Indent"=2, "Can Read?"=TRUE, "Can Write?"=TRUE, "Is Read?"=FALSE, "Is Write?"=FALSE, "Inactive Parent?"=FALSE, "Unwired?"=FALSE}, {"Label"="Visible", "Tag"="182,1,MCListbox (strict),6332005.632cc06,Label.Visible", "Property Type"=enum."Base", "Indent"=1, "Can Read?"=TRUE, "Can Write?"=TRUE, "Is Read?"=FALSE, "Is Write?"=FALSE, "Inactive Parent?"=FALSE, "Unwired?"=FALSE}, {"Label"="Attached Object", "Tag"="183,1,MCListbox (strict),6332005.632d819,Label.Attached Object", "Property Type"=enum."Base", "Indent"=1, "Can Read?"=TRUE, "Can Write?"=TRUE, "Is Read?"=FALSE, "Is Write?"=FALSE, "Inactive Parent?"=FALSE, "Unwired?"=FALSE}, {"Label"="Document Bounds", "Tag"="184,2,MCListbox (strict),6332005.632d812,Label.Document Bounds", "Property Type"=enum."Scripting", "Indent"=1, "Can Read?"=TRUE, "Can Write?"=FALSE, "Is Read?"=FALSE, "Is Write?"=FALSE, "Inactive Parent?"=FALSE, "Unwired?"=FALSE}, {"Label"="Height", "Tag"="185,2,MCListbox (strict),6332005.632d814,Label.Document Bounds:Height", "Property Type"=enum."Scripting", "Indent"=2, "Can Read?"=TRUE, "Can Write?"=FALSE, "Is Read?"=FALSE, "Is Write?"=FALSE, "Inactive Parent?"=FALSE, "Unwired?"=FALSE}, {"Label"="Width", "Tag"="186,2,MCListbox (strict),6332005.632d813,Label.Document Bounds:Width", "Property Type"=enum."Scripting", "Indent"=2, "Can Read?"=TRUE, "Can Write?"=FALSE, "Is Read?"=FALSE, "Is Write?"=FALSE, "Inactive Parent?"=FALSE, "Unwired?"=FALSE}, {"Label"="Enable Hyperlinks", "Tag"="187,1,MCListbox (strict),6332005.632d81a,Label.Enable Hyperlinks", "Property Type"=enum."Base", "Indent"=1, "Can Read?"=TRUE, "Can Write?"=TRUE, "Is Read?"=FALSE, "Is Write?"=FALSE, "Inactive Parent?"=FALSE, "Unwired?"=FALSE}, {"Label"="Font", "Tag"="188,1,MCListbox (strict),6332005.632d801,Label.Font", "Property Type"=enum."Base", "Indent"=1, "Can Read?"=TRUE, "Can Write?"=TRUE, "Is Read?"=FALSE, "Is Write?"=FALSE, "Inactive Parent?"=FALSE, "Unwired?"=FALSE}, {"Label"="Bold", "Tag"="189,1,MCListbox (strict),6332005.632d809,Label.Font:Bold", "Property Type"=enum."Base", "Indent"=2, "Can Read?"=TRUE, "Can Write?"=TRUE, "Is Read?"=FALSE, "Is Write?"=FALSE, "Inactive Parent?"=FALSE, "Unwired?"=FALSE}, {"Label"="Color", "Tag"="190,1,MCListbox (strict),6332005.632d80d,Label.Font:Color", "Property Type"=enum."Base", "Indent"=2, "Can Read?"=TRUE, "Can Write?"=TRUE, "Is Read?"=FALSE, "Is Write?"=FALSE, "Inactive Parent?"=FALSE, "Unwired?"=FALSE}, {"Label"="Italic", "Tag"="191,1,MCListbox (strict),6332005.632d80a,Label.Font:Italic", "Property Type"=enum."Base", "Indent"=2, "Can Read?"=TRUE, "Can Write?"=TRUE, "Is Read?"=FALSE, "Is Write?"=FALSE, "Inactive Parent?"=FALSE, "Unwired?"=FALSE}, {"Label"="Name", "Tag"="192,1,MCListbox (strict),6332005.632d807,Label.Font:Name", "Property Type"=enum."Base", "Indent"=2, "Can Read?"=TRUE, "Can Write?"=TRUE, "Is Read?"=FALSE, "Is Write?"=FALSE, "Inactive Parent?"=FALSE, "Unwired?"=FALSE}, {"Label"="Size", "Tag"="193,1,MCListbox (strict),6332005.632d808,Label.Font:Size", "Property Type"=enum."Base", "Indent"=2, "Can Read?"=TRUE, "Can Write?"=TRUE, "Is Read?"=FALSE, "Is Write?"=FALSE, "Inactive Parent?"=FALSE, "Unwired?"=FALSE}, {"Label"="Strikeout", "Tag"="194,1,MCListbox (strict),6332005.632d80c,Label.Font:Strikeout", "Property Type"=enum."Base", "Indent"=2, "Can Read?"=TRUE, "Can Write?"=TRUE, "Is Read?"=FALSE, "Is Write?"=FALSE, "Inactive Parent?"=FALSE, "Unwired?"=FALSE}, {"Label"="Underline", "Tag"="195,1,MCListbox (strict),6332005.632d80b,Label.Font:Underline", "Property Type"=enum."Base", "Indent"=2, "Can Read?"=TRUE, "Can Write?"=TRUE, "Is Read?"=FALSE, "Is Write?"=FALSE, "Inactive Parent?"=FALSE, "Unwired?"=FALSE}, {"Label"="FontType", "Tag"="196,3,MCListbox (strict),6332005.632d818,Label.FontType", "Property Type"=enum."Private", "Indent"=1, "Can Read?"=FALSE, "Can Write?"=TRUE, "Is Read?"=FALSE, "Is Write?"=FALSE, "Inactive Parent?"=FALSE, "Unwired?"=FALSE}, {"Label"="Interpret As Unicode", "Tag"="197,3,MCListbox (strict),6332005.632d811,Label.Interpret As Unicode", "Property Type"=enum."Private", "Indent"=1, "Can Read?"=TRUE, "Can Write?"=TRUE, "Is Read?"=FALSE, "Is Write?"=FALSE, "Inactive Parent?"=FALSE, "Unwired?"=FALSE}, {"Label"="Justification", "Tag"="198,1,MCListbox (strict),6332005.632d815,Label.Justification", "Property Type"=enum."Base", "Indent"=1, "Can Read?"=TRUE, "Can Write?"=TRUE, "Is Read?"=FALSE, "Is Write?"=FALSE, "Inactive Parent?"=FALSE, "Unwired?"=FALSE}, {"Label"="Lock", "Tag"="199,1,MCListbox (strict),6332005.632d817,Label.Lock", "Property Type"=enum."Base", "Indent"=1, "Can Read?"=TRUE, "Can Write?"=TRUE, "Is Read?"=FALSE, "Is Write?"=FALSE, "Inactive Parent?"=FALSE, "Unwired?"=FALSE}, {"Label"="Scroll Position", "Tag"="200,1,MCListbox (strict),6332005.632d805,Label.Scroll Position", "Property Type"=enum."Base", "Indent"=1, "Can Read?"=TRUE, "Can Write?"=TRUE, "Is Read?"=FALSE, "Is Write?"=FALSE, "Inactive Parent?"=FALSE, "Unwired?"=FALSE}, {"Label"="Selection", "Tag"="201,1,MCListbox (strict),6332005.632d802,Label.Selection", "Property Type"=enum."Base", "Indent"=1, "Can Read?"=TRUE, "Can Write?"=TRUE, "Is Read?"=FALSE, "Is Write?"=FALSE, "Inactive Parent?"=FALSE, "Unwired?"=FALSE}, {"Label"="End", "Tag"="202,1,MCListbox (strict),6332005.632d804,Label.Selection:End", "Property Type"=enum."Base", "Indent"=2, "Can Read?"=TRUE, "Can Write?"=TRUE, "Is Read?"=FALSE, "Is Write?"=FALSE, "Inactive Parent?"=FALSE, "Unwired?"=FALSE}, {"Label"="Start", "Tag"="203,1,MCListbox (strict),6332005.632d803,Label.Selection:Start", "Property Type"=enum."Base", "Indent"=2, "Can Read?"=TRUE, "Can Write?"=TRUE, "Is Read?"=FALSE, "Is Write?"=FALSE, "Inactive Parent?"=FALSE, "Unwired?"=FALSE}, {"Label"="Size to Text?", "Tag"="204,1,MCListbox (strict),6332005.632d806,Label.Size to Text?", "Property Type"=enum."Base", "Indent"=1, "Can Read?"=TRUE, "Can Write?"=TRUE, "Is Read?"=FALSE, "Is Write?"=FALSE, "Inactive Parent?"=FALSE, "Unwired?"=FALSE}, {"Label"="Text", "Tag"="205,1,MCListbox (strict),6332005.632d800,Label.Text", "Property Type"=enum."Base", "Indent"=1, "Can Read?"=TRUE, "Can Write?"=TRUE, "Is Read?"=FALSE, "Is Write?"=FALSE, "Inactive Parent?"=FALSE, "Unwired?"=FALSE}, {"Label"="Text Colors", "Tag"="206,1,MCListbox (strict),6332005.632d80e,Label.Text Colors", "Property Type"=enum."Base", "Indent"=1, "Can Read?"=TRUE, "Can Write?"=TRUE, "Is Read?"=FALSE, "Is Write?"=FALSE, "Inactive Parent?"=FALSE, "Unwired?"=FALSE}, {"Label"="BG Color", "Tag"="207,1,MCListbox (strict),6332005.632d810,Label.Text Colors:BG Color", "Property Type"=enum."Base", "Indent"=2, "Can Read?"=TRUE, "Can Write?"=TRUE, "Is Read?"=FALSE, "Is Write?"=FALSE, "Inactive Parent?"=FALSE, "Unwired?"=FALSE}, {"Label"="Text Color", "Tag"="208,1,MCListbox (strict),6332005.632d80f,Label.Text Colors:Text Color", "Property Type"=enum."Base", "Indent"=2, "Can Read?"=TRUE, "Can Write?"=TRUE, "Is Read?"=FALSE, "Is Write?"=FALSE, "Inactive Parent?"=FALSE, "Unwired?"=FALSE}, {"Label"="Text Overflow", "Tag"="209,1,MCListbox (strict),6332005.632d81b,Label.Text Overflow", "Property Type"=enum."Base", "Indent"=1, "Can Read?"=TRUE, "Can Write?"=TRUE, "Is Read?"=FALSE, "Is Write?"=FALSE, "Inactive Parent?"=FALSE, "Unwired?"=FALSE}, {"Label"="Vertical Arrangement", "Tag"="210,1,MCListbox (strict),6332005.632d816,Label.Vertical Arrangement", "Property Type"=enum."Base", "Indent"=1, "Can Read?"=TRUE, "Can Write?"=TRUE, "Is Read?"=FALSE, "Is Write?"=FALSE, "Inactive Parent?"=FALSE, "Unwired?"=FALSE}, {"Label"="Latch Value", "Tag"="211,3,MCListbox (strict),633201f,Latch Value", "Property Type"=enum."Private", "Indent"=0, "Can Read?"=TRUE, "Can Write?"=TRUE, "Is Read?"=FALSE, "Is Write?"=FALSE, "Inactive Parent?"=FALSE, "Unwired?"=FALSE}, {"Label"="Local Variables[]", "Tag"="212,2,MCListbox (strict),633200a,Local Variables[]", "Property Type"=enum."Scripting", "Indent"=0, "Can Read?"=TRUE, "Can Write?"=FALSE, "Is Read?"=FALSE, "Is Write?"=FALSE, "Inactive Parent?"=FALSE, "Unwired?"=FALSE}, {"Label"="Owning Pane", "Tag"="213,1,MCListbox (strict),633203e,Owning Pane", "Property Type"=enum."Base", "Indent"=0, "Can Read?"=TRUE, "Can Write?"=FALSE, "Is Read?"=FALSE, "Is Write?"=FALSE, "Inactive Parent?"=FALSE, "Unwired?"=FALSE}, {"Label"="Property Nodes[]", "Tag"="214,2,MCListbox (strict),633200b,Property Nodes[]", "Property Type"=enum."Scripting", "Indent"=0, "Can Read?"=TRUE, "Can Write?"=FALSE, "Is Read?"=FALSE, "Is Write?"=FALSE, "Inactive Parent?"=FALSE, "Unwired?"=FALSE}, {"Label"="Skip When Tabbing", "Tag"="215,1,MCListbox (strict),6332021,Skip When Tabbing", "Property Type"=enum."Base", "Indent"=0, "Can Read?"=TRUE, "Can Write?"=TRUE, "Is Read?"=FALSE, "Is Write?"=FALSE, "Inactive Parent?"=FALSE, "Unwired?"=FALSE}, {"Label"="Style ID", "Tag"="216,2,MCListbox (strict),633203a,Style ID", "Property Type"=enum."Scripting", "Indent"=0, "Can Read?"=TRUE, "Can Write?"=FALSE, "Is Read?"=FALSE, "Is Write?"=FALSE, "Inactive Parent?"=FALSE, "Unwired?"=FALSE}, {"Label"="Synchronous Display", "Tag"="217,1,MCListbox (strict),6332008,Synchronous Display", "Property Type"=enum."Base", "Indent"=0, "Can Read?"=TRUE, "Can Write?"=TRUE, "Is Read?"=FALSE, "Is Write?"=FALSE, "Inactive Parent?"=FALSE, "Unwired?"=FALSE}, {"Label"="Terminal", "Tag"="218,2,MCListbox (strict),6332006,Terminal", "Property Type"=enum."Scripting", "Indent"=0, "Can Read?"=TRUE, "Can Write?"=FALSE, "Is Read?"=FALSE, "Is Write?"=FALSE, "Inactive Parent?"=FALSE, "Unwired?"=FALSE}, {"Label"="Tip Strip", "Tag"="219,1,MCListbox (strict),6332014,Tip Strip", "Property Type"=enum."Base", "Indent"=0, "Can Read?"=TRUE, "Can Write?"=TRUE, "Is Read?"=FALSE, "Is Write?"=FALSE, "Inactive Parent?"=FALSE, "Unwired?"=FALSE}, {"Label"="Typedef", "Tag"="220,2,MCListbox (strict),633201b,Typedef", "Property Type"=enum."None", "Indent"=0, "Can Read?"=FALSE, "Can Write?"=FALSE, "Is Read?"=FALSE, "Is Write?"=FALSE, "Inactive Parent?"=TRUE, "Unwired?"=FALSE}, {"Label"="Path", "Tag"="221,2,MCListbox (strict),633201b,Typedef:Path", "Property Type"=enum."Scripting", "Indent"=1, "Can Read?"=TRUE, "Can Write?"=FALSE, "Is Read?"=FALSE, "Is Write?"=FALSE, "Inactive Parent?"=FALSE, "Unwired?"=FALSE}, {"Label"="VI", "Tag"="222,2,MCListbox (strict),6332025,Typedef:VI", "Property Type"=enum."Scripting", "Indent"=1, "Can Read?"=TRUE, "Can Write?"=FALSE, "Is Read?"=FALSE, "Is Write?"=FALSE, "Inactive Parent?"=FALSE, "Unwired?"=FALSE}, {"Label"="Value", "Tag"="223,1,MCListbox (strict),6332012,Value", "Property Type"=enum."Base", "Indent"=0, "Can Read?"=TRUE, "Can Write?"=TRUE, "Is Read?"=FALSE, "Is Write?"=FALSE, "Inactive Parent?"=FALSE, "Unwired?"=FALSE}, {"Label"="Value (Signaling)", "Tag"="224,1,MCListbox (strict),6332024,Value (Signaling)", "Property Type"=enum."Base", "Indent"=0, "Can Read?"=FALSE, "Can Write?"=TRUE, "Is Read?"=FALSE, "Is Write?"=FALSE, "Inactive Parent?"=FALSE, "Unwired?"=FALSE}, {"Label"="Value (Undoable)", "Tag"="225,2,MCListbox (strict),6332041,Value (Undoable)", "Property Type"=enum."Scripting", "Indent"=0, "Can Read?"=FALSE, "Can Write?"=TRUE, "Is Read?"=FALSE, "Is Write?"=FALSE, "Inactive Parent?"=FALSE, "Unwired?"=FALSE}, {"Label"="Visible", "Tag"="226,1,MCListbox (strict),6332000,Visible", "Property Type"=enum."Base", "Indent"=0, "Can Read?"=TRUE, "Can Write?"=TRUE, "Is Read?"=FALSE, "Is Write?"=FALSE, "Inactive Parent?"=FALSE, "Unwired?"=FALSE}, {"Label"="Wizard Data", "Tag"="227,3,MCListbox (strict),6332019,Wizard Data", "Property Type"=enum."Private", "Indent"=0, "Can Read?"=TRUE, "Can Write?"=TRUE, "Is Read?"=FALSE, "Is Write?"=FALSE, "Inactive Parent?"=FALSE, "Unwired?"=FALSE}, {"Label"="XControl", "Tag"="228,1,MCListbox (strict),6332037,XControl", "Property Type"=enum."None", "Indent"=0, "Can Read?"=FALSE, "Can Write?"=FALSE, "Is Read?"=FALSE, "Is Write?"=FALSE, "Inactive Parent?"=TRUE, "Unwired?"=FALSE}, {"Label"="Container Bounds", "Tag"="229,1,MCListbox (strict),6332037,XControl:Container Bounds", "Property Type"=enum."Base", "Indent"=1, "Can Read?"=TRUE, "Can Write?"=TRUE, "Is Read?"=FALSE, "Is Write?"=FALSE, "Inactive Parent?"=FALSE, "Unwired?"=FALSE}, {"Label"="Container Bounds:Height", "Tag"="230,1,MCListbox (strict),6332039,XControl:Container Bounds:Height", "Property Type"=enum."Base", "Indent"=2, "Can Read?"=TRUE, "Can Write?"=TRUE, "Is Read?"=FALSE, "Is Write?"=FALSE, "Inactive Parent?"=FALSE, "Unwired?"=FALSE}, {"Label"="Container Bounds:Width", "Tag"="231,1,MCListbox (strict),6332038,XControl:Container Bounds:Width", "Property Type"=enum."Base", "Indent"=2, "Can Read?"=TRUE, "Can Write?"=TRUE, "Is Read?"=FALSE, "Is Write?"=FALSE, "Inactive Parent?"=FALSE, "Unwired?"=FALSE}, {"Label"="Is XControl?", "Tag"="232,1,MCListbox (strict),6332036,XControl:Is XControl?", "Property Type"=enum."Base", "Indent"=1, "Can Read?"=TRUE, "Can Write?"=FALSE, "Is Read?"=FALSE, "Is Write?"=FALSE, "Inactive Parent?"=FALSE, "Unwired?"=FALSE}, {"Label"="Divider", "Tag"="233,6,MCListbox (strict),Divider,Divider", "Property Type"=enum."Divider", "Indent"=0, "Can Read?"=FALSE, "Can Write?"=FALSE, "Is Read?"=FALSE, "Is Write?"=FALSE, "Inactive Parent?"=FALSE, "Unwired?"=FALSE}, {"Label"="Active Cell", "Tag"="234,1,MCListbox (strict),18d9900e,Active Cell", "Property Type"=enum."None", "Indent"=0, "Can Read?"=FALSE, "Can Write?"=FALSE, "Is Read?"=FALSE, "Is Write?"=FALSE, "Inactive Parent?"=TRUE, "Unwired?"=FALSE}, {"Label"="Active Cell", "Tag"="235,1,MCListbox (strict),18d9900e,Active Cell:Active Cell", "Property Type"=enum."Base", "Indent"=1, "Can Read?"=TRUE, "Can Write?"=TRUE, "Is Read?"=FALSE, "Is Write?"=FALSE, "Inactive Parent?"=FALSE, "Unwired?"=FALSE}, {"Label"="Cell Background Color", "Tag"="236,1,MCListbox (strict),18d99010,Active Cell:Cell Background Color", "Property Type"=enum."Base", "Indent"=1, "Can Read?"=TRUE, "Can Write?"=TRUE, "Is Read?"=FALSE, "Is Write?"=FALSE, "Inactive Parent?"=FALSE, "Unwired?"=FALSE}, {"Label"="Cell Font", "Tag"="237,1,MCListbox (strict),18d99025,Active Cell:Cell Font", "Property Type"=enum."Base", "Indent"=1, "Can Read?"=TRUE, "Can Write?"=TRUE, "Is Read?"=FALSE, "Is Write?"=FALSE, "Inactive Parent?"=FALSE, "Unwired?"=FALSE}, {"Label"="Cell Font:Bold", "Tag"="238,1,MCListbox (strict),18d99028,Active Cell:Cell Font:Bold", "Property Type"=enum."Base", "Indent"=2, "Can Read?"=TRUE, "Can Write?"=TRUE, "Is Read?"=FALSE, "Is Write?"=FALSE, "Inactive Parent?"=FALSE, "Unwired?"=FALSE}, {"Label"="Cell Font:Color", "Tag"="239,1,MCListbox (strict),18d9902c,Active Cell:Cell Font:Color", "Property Type"=enum."Base", "Indent"=2, "Can Read?"=TRUE, "Can Write?"=TRUE, "Is Read?"=FALSE, "Is Write?"=FALSE, "Inactive Parent?"=FALSE, "Unwired?"=FALSE}, {"Label"="Cell Font:Italic", "Tag"="240,1,MCListbox (strict),18d99029,Active Cell:Cell Font:Italic", "Property Type"=enum."Base", "Indent"=2, "Can Read?"=TRUE, "Can Write?"=TRUE, "Is Read?"=FALSE, "Is Write?"=FALSE, "Inactive Parent?"=FALSE, "Unwired?"=FALSE}, {"Label"="Cell Font:Name", "Tag"="241,1,MCListbox (strict),18d99026,Active Cell:Cell Font:Name", "Property Type"=enum."Base", "Indent"=2, "Can Read?"=TRUE, "Can Write?"=TRUE, "Is Read?"=FALSE, "Is Write?"=FALSE, "Inactive Parent?"=FALSE, "Unwired?"=FALSE}, {"Label"="Cell Font:Size", "Tag"="242,1,MCListbox (strict),18d99027,Active Cell:Cell Font:Size", "Property Type"=enum."Base", "Indent"=2, "Can Read?"=TRUE, "Can Write?"=TRUE, "Is Read?"=FALSE, "Is Write?"=FALSE, "Inactive Parent?"=FALSE, "Unwired?"=FALSE}, {"Label"="Cell Font:Strikeout", "Tag"="243,1,MCListbox (strict),18d9902b,Active Cell:Cell Font:Strikeout", "Property Type"=enum."Base", "Indent"=2, "Can Read?"=TRUE, "Can Write?"=TRUE, "Is Read?"=FALSE, "Is Write?"=FALSE, "Inactive Parent?"=FALSE, "Unwired?"=FALSE}, {"Label"="Cell Font:Underline", "Tag"="244,1,MCListbox (strict),18d9902a,Active Cell:Cell Font:Underline", "Property Type"=enum."Base", "Indent"=2, "Can Read?"=TRUE, "Can Write?"=TRUE, "Is Read?"=FALSE, "Is Write?"=FALSE, "Inactive Parent?"=FALSE, "Unwired?"=FALSE}, {"Label"="Cell Justification", "Tag"="245,1,MCListbox (strict),18d9902d,Active Cell:Cell Justification", "Property Type"=enum."Base", "Indent"=1, "Can Read?"=TRUE, "Can Write?"=TRUE, "Is Read?"=FALSE, "Is Write?"=FALSE, "Inactive Parent?"=FALSE, "Unwired?"=FALSE}, {"Label"="Cell Size", "Tag"="246,1,MCListbox (strict),18d99011,Active Cell:Cell Size", "Property Type"=enum."Base", "Indent"=1, "Can Read?"=TRUE, "Can Write?"=TRUE, "Is Read?"=FALSE, "Is Write?"=FALSE, "Inactive Parent?"=FALSE, "Unwired?"=FALSE}, {"Label"="Cell Size:Height", "Tag"="247,1,MCListbox (strict),18d99013,Active Cell:Cell Size:Height", "Property Type"=enum."Base", "Indent"=2, "Can Read?"=TRUE, "Can Write?"=TRUE, "Is Read?"=FALSE, "Is Write?"=FALSE, "Inactive Parent?"=FALSE, "Unwired?"=FALSE}, {"Label"="Cell Size:Width", "Tag"="248,1,MCListbox (strict),18d99012,Active Cell:Cell Size:Width", "Property Type"=enum."Base", "Indent"=2, "Can Read?"=TRUE, "Can Write?"=TRUE, "Is Read?"=FALSE, "Is Write?"=FALSE, "Inactive Parent?"=FALSE, "Unwired?"=FALSE}, {"Label"="Position", "Tag"="249,1,MCListbox (strict),18d99022,Active Cell:Position", "Property Type"=enum."Base", "Indent"=1, "Can Read?"=TRUE, "Can Write?"=FALSE, "Is Read?"=FALSE, "Is Write?"=FALSE, "Inactive Parent?"=FALSE, "Unwired?"=FALSE}, {"Label"="Position:Left", "Tag"="250,1,MCListbox (strict),18d99023,Active Cell:Position:Left", "Property Type"=enum."Base", "Indent"=2, "Can Read?"=TRUE, "Can Write?"=FALSE, "Is Read?"=FALSE, "Is Write?"=FALSE, "Inactive Parent?"=FALSE, "Unwired?"=FALSE}, {"Label"="Position:Top", "Tag"="251,1,MCListbox (strict),18d99024,Active Cell:Position:Top", "Property Type"=enum."Base", "Indent"=2, "Can Read?"=TRUE, "Can Write?"=FALSE, "Is Read?"=FALSE, "Is Write?"=FALSE, "Inactive Parent?"=FALSE, "Unwired?"=FALSE}, {"Label"="Allow Editing Cells", "Tag"="252,1,MCListbox (strict),18d9902f,Allow Editing Cells", "Property Type"=enum."Base", "Indent"=0, "Can Read?"=TRUE, "Can Write?"=TRUE, "Is Read?"=FALSE, "Is Write?"=FALSE, "Inactive Parent?"=FALSE, "Unwired?"=FALSE}, {"Label"="Autosizing Row Height", "Tag"="253,1,MCListbox (strict),18d99015,Autosizing Row Height", "Property Type"=enum."Base", "Indent"=0, "Can Read?"=TRUE, "Can Write?"=TRUE, "Is Read?"=FALSE, "Is Write?"=FALSE, "Inactive Parent?"=FALSE, "Unwired?"=FALSE}, {"Label"="Bulk Cells", "Tag"="254,3,MCListbox (strict),18d9903e,Bulk Cells", "Property Type"=enum."None", "Indent"=0, "Can Read?"=FALSE, "Can Write?"=FALSE, "Is Read?"=FALSE, "Is Write?"=FALSE, "Inactive Parent?"=TRUE, "Unwired?"=FALSE}, {"Label"="Background Color", "Tag"="255,3,MCListbox (strict),18d9903e,Bulk Cells:Background Color", "Property Type"=enum."Private", "Indent"=1, "Can Read?"=FALSE, "Can Write?"=TRUE, "Is Read?"=FALSE, "Is Write?"=FALSE, "Inactive Parent?"=FALSE, "Unwired?"=FALSE}, {"Label"="Font Color", "Tag"="256,3,MCListbox (strict),18d9903f,Bulk Cells:Font Color", "Property Type"=enum."Private", "Indent"=1, "Can Read?"=FALSE, "Can Write?"=TRUE, "Is Read?"=FALSE, "Is Write?"=FALSE, "Inactive Parent?"=FALSE, "Unwired?"=FALSE}, {"Label"="Column Header Strings[]", "Tag"="257,1,MCListbox (strict),18d99005,Column Header Strings[]", "Property Type"=enum."Base", "Indent"=0, "Can Read?"=TRUE, "Can Write?"=TRUE, "Is Read?"=FALSE, "Is Write?"=FALSE, "Inactive Parent?"=FALSE, "Unwired?"=FALSE}, {"Label"="Content Rect Bounds", "Tag"="258,1,MCListbox (strict),18d9901f,Content Rect Bounds", "Property Type"=enum."Base", "Indent"=0, "Can Read?"=TRUE, "Can Write?"=FALSE, "Is Read?"=FALSE, "Is Write?"=FALSE, "Inactive Parent?"=FALSE, "Unwired?"=FALSE}, {"Label"="Height", "Tag"="259,1,MCListbox (strict),18d99021,Content Rect Bounds:Height", "Property Type"=enum."Base", "Indent"=1, "Can Read?"=TRUE, "Can Write?"=FALSE, "Is Read?"=FALSE, "Is Write?"=FALSE, "Inactive Parent?"=FALSE, "Unwired?"=FALSE}, {"Label"="Width", "Tag"="260,1,MCListbox (strict),18d99020,Content Rect Bounds:Width", "Property Type"=enum."Base", "Indent"=1, "Can Read?"=TRUE, "Can Write?"=FALSE, "Is Read?"=FALSE, "Is Write?"=FALSE, "Inactive Parent?"=FALSE, "Unwired?"=FALSE}, {"Label"="Content Rect Position", "Tag"="261,1,MCListbox (strict),18d9901c,Content Rect Position", "Property Type"=enum."Base", "Indent"=0, "Can Read?"=TRUE, "Can Write?"=FALSE, "Is Read?"=FALSE, "Is Write?"=FALSE, "Inactive Parent?"=FALSE, "Unwired?"=FALSE}, {"Label"="Left", "Tag"="262,1,MCListbox (strict),18d9901d,Content Rect Position:Left", "Property Type"=enum."Base", "Indent"=1, "Can Read?"=TRUE, "Can Write?"=FALSE, "Is Read?"=FALSE, "Is Write?"=FALSE, "Inactive Parent?"=FALSE, "Unwired?"=FALSE}, {"Label"="Top", "Tag"="263,1,MCListbox (strict),18d9901e,Content Rect Position:Top", "Property Type"=enum."Base", "Indent"=1, "Can Read?"=TRUE, "Can Write?"=FALSE, "Is Read?"=FALSE, "Is Write?"=FALSE, "Inactive Parent?"=FALSE, "Unwired?"=FALSE}, {"Label"="Disabled Items", "Tag"="264,1,MCListbox (strict),18d99002,Disabled Items", "Property Type"=enum."Base", "Indent"=0, "Can Read?"=TRUE, "Can Write?"=TRUE, "Is Read?"=FALSE, "Is Write?"=FALSE, "Inactive Parent?"=FALSE, "Unwired?"=FALSE}, {"Label"="Drag/Drop", "Tag"="265,1,MCListbox (strict),18d9903a,Drag/Drop", "Property Type"=enum."None", "Indent"=0, "Can Read?"=FALSE, "Can Write?"=FALSE, "Is Read?"=FALSE, "Is Write?"=FALSE, "Inactive Parent?"=TRUE, "Unwired?"=FALSE}, {"Label"="Allow Drag and Drop Outside Control", "Tag"="266,1,MCListbox (strict),18d9903a,Drag/Drop:Allow Drag and Drop Outside Control", "Property Type"=enum."Base", "Indent"=1, "Can Read?"=TRUE, "Can Write?"=TRUE, "Is Read?"=FALSE, "Is Write?"=FALSE, "Inactive Parent?"=FALSE, "Unwired?"=FALSE}, {"Label"="Allow Dragging", "Tag"="267,1,MCListbox (strict),18d99037,Drag/Drop:Allow Dragging", "Property Type"=enum."Base", "Indent"=1, "Can Read?"=TRUE, "Can Write?"=TRUE, "Is Read?"=FALSE, "Is Write?"=FALSE, "Inactive Parent?"=FALSE, "Unwired?"=FALSE}, {"Label"="Allow Dropping", "Tag"="268,1,MCListbox (strict),18d99038,Drag/Drop:Allow Dropping", "Property Type"=enum."Base", "Indent"=1, "Can Read?"=TRUE, "Can Write?"=TRUE, "Is Read?"=FALSE, "Is Write?"=FALSE, "Inactive Parent?"=FALSE, "Unwired?"=FALSE}, {"Label"="Drag Mode", "Tag"="269,1,MCListbox (strict),18d99039,Drag/Drop:Drag Mode", "Property Type"=enum."Base", "Indent"=1, "Can Read?"=TRUE, "Can Write?"=TRUE, "Is Read?"=FALSE, "Is Write?"=FALSE, "Inactive Parent?"=FALSE, "Unwired?"=FALSE}, {"Label"="Edit Position", "Tag"="270,1,MCListbox (strict),18d9903c,Edit Position", "Property Type"=enum."Base", "Indent"=0, "Can Read?"=TRUE, "Can Write?"=TRUE, "Is Read?"=FALSE, "Is Write?"=FALSE, "Inactive Parent?"=FALSE, "Unwired?"=FALSE}, {"Label"="Focus Row", "Tag"="271,1,MCListbox (strict),18d9903d,Focus Row", "Property Type"=enum."Base", "Indent"=0, "Can Read?"=TRUE, "Can Write?"=TRUE, "Is Read?"=FALSE, "Is Write?"=FALSE, "Inactive Parent?"=FALSE, "Unwired?"=FALSE}, {"Label"="Is Array?", "Tag"="272,2,MCListbox (strict),18d99033,Is Array?", "Property Type"=enum."Scripting", "Indent"=0, "Can Read?"=TRUE, "Can Write?"=TRUE, "Is Read?"=FALSE, "Is Write?"=FALSE, "Inactive Parent?"=FALSE, "Unwired?"=FALSE}, {"Label"="Item Names", "Tag"="273,1,MCListbox (strict),18d99000,Item Names", "Property Type"=enum."Base", "Indent"=0, "Can Read?"=TRUE, "Can Write?"=TRUE, "Is Read?"=FALSE, "Is Write?"=FALSE, "Inactive Parent?"=FALSE, "Unwired?"=FALSE}, {"Label"="Item Symbols", "Tag"="274,1,MCListbox (strict),18d99001,Item Symbols", "Property Type"=enum."Base", "Indent"=0, "Can Read?"=TRUE, "Can Write?"=TRUE, "Is Read?"=FALSE, "Is Write?"=FALSE, "Inactive Parent?"=FALSE, "Unwired?"=FALSE}, {"Label"="Keyboard Mode", "Tag"="275,1,MCListbox (strict),18d99034,Keyboard Mode", "Property Type"=enum."Base", "Indent"=0, "Can Read?"=TRUE, "Can Write?"=TRUE, "Is Read?"=FALSE, "Is Write?"=FALSE, "Inactive Parent?"=FALSE, "Unwired?"=FALSE}, {"Label"="Multiple Line Input", "Tag"="276,1,MCListbox (strict),18d99017,Multiple Line Input", "Property Type"=enum."Base", "Indent"=0, "Can Read?"=TRUE, "Can Write?"=TRUE, "Is Read?"=FALSE, "Is Write?"=FALSE, "Inactive Parent?"=FALSE, "Unwired?"=FALSE}, {"Label"="Number of Columns", "Tag"="277,1,MCListbox (strict),18d9900a,Number of Columns", "Property Type"=enum."Base", "Indent"=0, "Can Read?"=TRUE, "Can Write?"=TRUE, "Is Read?"=FALSE, "Is Write?"=FALSE, "Inactive Parent?"=FALSE, "Unwired?"=FALSE}, {"Label"="Number of Rows", "Tag"="278,1,MCListbox (strict),18d99009,Number of Rows", "Property Type"=enum."Base", "Indent"=0, "Can Read?"=TRUE, "Can Write?"=TRUE, "Is Read?"=FALSE, "Is Write?"=FALSE, "Inactive Parent?"=FALSE, "Unwired?"=FALSE}, {"Label"="Row Header Strings[]", "Tag"="279,1,MCListbox (strict),18d99032,Row Header Strings[]", "Property Type"=enum."Base", "Indent"=0, "Can Read?"=TRUE, "Can Write?"=TRUE, "Is Read?"=FALSE, "Is Write?"=FALSE, "Inactive Parent?"=FALSE, "Unwired?"=FALSE}, {"Label"="Select Entire Rows", "Tag"="280,2,MCListbox (strict),18d9903b,Select Entire Rows", "Property Type"=enum."Scripting", "Indent"=0, "Can Read?"=TRUE, "Can Write?"=TRUE, "Is Read?"=FALSE, "Is Write?"=FALSE, "Inactive Parent?"=FALSE, "Unwired?"=FALSE}, {"Label"="Selected Cell", "Tag"="281,3,MCListbox (strict),18d99018,Selected Cell", "Property Type"=enum."Private", "Indent"=0, "Can Read?"=TRUE, "Can Write?"=TRUE, "Is Read?"=FALSE, "Is Write?"=FALSE, "Inactive Parent?"=FALSE, "Unwired?"=FALSE}, {"Label"="Selection Color", "Tag"="282,1,MCListbox (strict),18d99014,Selection Color", "Property Type"=enum."Base", "Indent"=0, "Can Read?"=TRUE, "Can Write?"=TRUE, "Is Read?"=FALSE, "Is Write?"=FALSE, "Inactive Parent?"=FALSE, "Unwired?"=FALSE}, {"Label"="Selection Mode", "Tag"="283,1,MCListbox (strict),18d9900d,Selection Mode", "Property Type"=enum."Base", "Indent"=0, "Can Read?"=TRUE, "Can Write?"=TRUE, "Is Read?"=FALSE, "Is Write?"=FALSE, "Inactive Parent?"=FALSE, "Unwired?"=FALSE}, {"Label"="Size", "Tag"="284,1,MCListbox (strict),18d99019,Size", "Property Type"=enum."Base", "Indent"=0, "Can Read?"=TRUE, "Can Write?"=TRUE, "Is Read?"=FALSE, "Is Write?"=FALSE, "Inactive Parent?"=FALSE, "Unwired?"=FALSE}, {"Label"="Height", "Tag"="285,1,MCListbox (strict),18d9901b,Size:Height", "Property Type"=enum."Base", "Indent"=1, "Can Read?"=TRUE, "Can Write?"=TRUE, "Is Read?"=FALSE, "Is Write?"=FALSE, "Inactive Parent?"=FALSE, "Unwired?"=FALSE}, {"Label"="Width", "Tag"="286,1,MCListbox (strict),18d9901a,Size:Width", "Property Type"=enum."Base", "Indent"=1, "Can Read?"=TRUE, "Can Write?"=TRUE, "Is Read?"=FALSE, "Is Write?"=FALSE, "Inactive Parent?"=FALSE, "Unwired?"=FALSE}, {"Label"="Smooth Horizontal Scrolling", "Tag"="287,1,MCListbox (strict),18d99016,Smooth Horizontal Scrolling", "Property Type"=enum."Base", "Indent"=0, "Can Read?"=TRUE, "Can Write?"=TRUE, "Is Read?"=FALSE, "Is Write?"=FALSE, "Inactive Parent?"=FALSE, "Unwired?"=FALSE}, {"Label"="Top Left Visible Cell", "Tag"="288,1,MCListbox (strict),18d9900c,Top Left Visible Cell", "Property Type"=enum."Base", "Indent"=0, "Can Read?"=TRUE, "Can Write?"=TRUE, "Is Read?"=FALSE, "Is Write?"=FALSE, "Inactive Parent?"=FALSE, "Unwired?"=FALSE}, {"Label"="Visible Items", "Tag"="289,1,MCListbox (strict),18d9900b,Visible Items", "Property Type"=enum."None", "Indent"=0, "Can Read?"=FALSE, "Can Write?"=FALSE, "Is Read?"=FALSE, "Is Write?"=FALSE, "Inactive Parent?"=TRUE, "Unwired?"=FALSE}, {"Label"="Column Headers Visible", "Tag"="290,1,MCListbox (strict),18d9900b,Visible Items:Column Headers Visible", "Property Type"=enum."Base", "Indent"=1, "Can Read?"=TRUE, "Can Write?"=TRUE, "Is Read?"=FALSE, "Is Write?"=FALSE, "Inactive Parent?"=FALSE, "Unwired?"=FALSE}, {"Label"="Horizontal Lines Visible", "Tag"="291,1,MCListbox (strict),18d99036,Visible Items:Horizontal Lines Visible", "Property Type"=enum."Base", "Indent"=1, "Can Read?"=TRUE, "Can Write?"=TRUE, "Is Read?"=FALSE, "Is Write?"=FALSE, "Inactive Parent?"=FALSE, "Unwired?"=FALSE}, {"Label"="Horizontal Scrollbar Visible", "Tag"="292,1,MCListbox (strict),18d99008,Visible Items:Horizontal Scrollbar Visible", "Property Type"=enum."Base", "Indent"=1, "Can Read?"=TRUE, "Can Write?"=TRUE, "Is Read?"=FALSE, "Is Write?"=FALSE, "Inactive Parent?"=FALSE, "Unwired?"=FALSE}, {"Label"="Row Headers Visible", "Tag"="293,1,MCListbox (strict),18d99031,Visible Items:Row Headers Visible", "Property Type"=enum."Base", "Indent"=1, "Can Read?"=TRUE, "Can Write?"=TRUE, "Is Read?"=FALSE, "Is Write?"=FALSE, "Inactive Parent?"=FALSE, "Unwired?"=FALSE}, {"Label"="Symbols Visible", "Tag"="294,1,MCListbox (strict),18d99006,Visible Items:Symbols Visible", "Property Type"=enum."Base", "Indent"=1, "Can Read?"=TRUE, "Can Write?"=TRUE, "Is Read?"=FALSE, "Is Write?"=FALSE, "Inactive Parent?"=FALSE, "Unwired?"=FALSE}, {"Label"="Vertical Lines Visible", "Tag"="295,1,MCListbox (strict),18d99035,Visible Items:Vertical Lines Visible", "Property Type"=enum."Base", "Indent"=1, "Can Read?"=TRUE, "Can Write?"=TRUE, "Is Read?"=FALSE, "Is Write?"=FALSE, "Inactive Parent?"=FALSE, "Unwired?"=FALSE}, {"Label"="Vertical Scrollbar Visible", "Tag"="296,1,MCListbox (strict),18d99007,Visible Items:Vertical Scrollbar Visible", "Property Type"=enum."Base", "Indent"=1, "Can Read?"=TRUE, "Can Write?"=TRUE, "Is Read?"=FALSE, "Is Write?"=FALSE, "Inactive Parent?"=FALSE, "Unwired?"=FALSE}]) -> (0 "Error Out":errorcluster, 2 "Placement Out":enum32{"Choice 1", "Choice 2"}(radio), 3 "Property Array Out":T3(array[cluster]))   [LabVIEW 2023]
doc: "Dialog to select items from the input cluster ref. \n\nFilter narrows list of items.\nDown key puts focus on tree and selects first item.\nUp and Down keps navigate tree.\nMultiple items can be selected.\n\nIn case of action \"Delete\" (\"Remove elements(s)...\" selected), list will show all elements currently displayed, else it will show all elements available to bundle or unbundle.\n\nOutput is a list of the selected item tags."
uses:
  controls/Done Button.ctl
  controls/action enum.ctl
  top/BundleMagic.ctl
panel:
  in  "Filter":string
  in  "Main Tree":string[](tree)
  in  "Write Tree":string[](tree)
  in  "Read Tree":string[](tree)
  out "Selected Element String":string
  in  "Boolean":bool
  in  "Property Display":T1
  in  "Placement":enum32{"Choice 1", "Choice 2"}(radio)
  in  "Done":T2
  in  "Show radio":bool
  # "#review need to place this string on GUI"
  # "Debug"
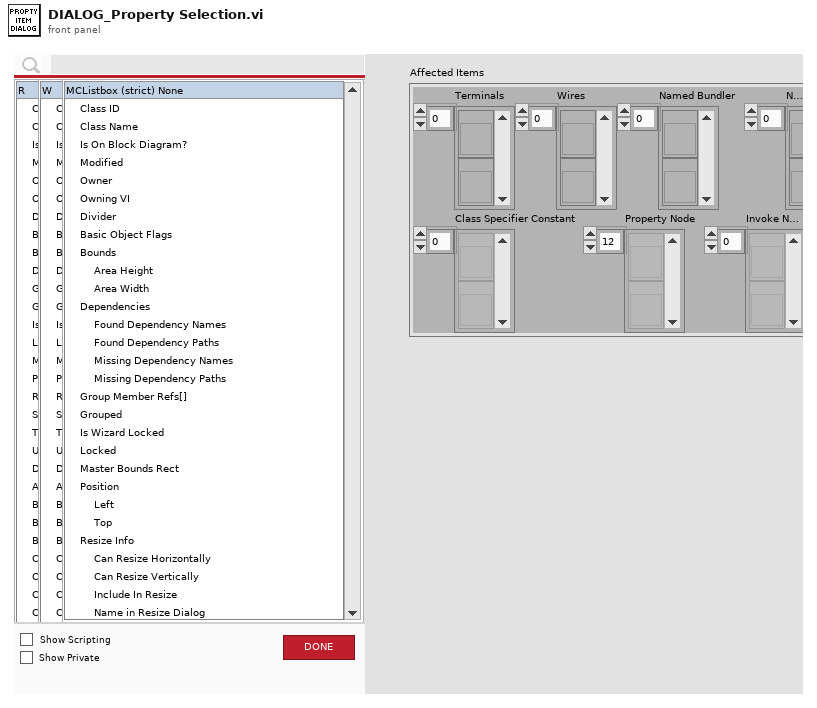
[diagram p1: front panel]
types:
  T1 = cluster{"Show Scripting":bool, "Show Private":bool}
  T2 = typedef "Done Button.ctl" = bool
  T3 = cluster{"Tag":string, "Read":bool, "Write":bool, "New":bool}[]
  T4 = typedef "BundleMagic.ctl" = cluster{"Terminals":refnum<vi>[], "Wires":refnum<vi>[], "Named Bundler":refnum<vi>[], "Named Unbundler":refnum<vi>[], "In Place Cluster Node":refnum<vi>[], "Class Specifier Constant":refnum<vi>[], "Property Node":refnum<vi>[], "Invoke Node":refnum<vi>[], "Refnum Control":refnum<vi>[]}
  T5 = cluster{"Label":string, "Tag":string, "Property Type":enum16{"Unknown", "Base", "Scripting", "Private", "Deprecated", "None", "Divider"}, "Indent":u16, "Can Read?":bool, "Can Write?":bool, "Is Read?":bool, "Is Write?":bool, "Inactive Parent?":bool, "Unwired?":bool}[]
  T6 = typedef "action enum.ctl" = enum16{"[NONE]", "Wire Bundle", "Wire Unbundle", "Terminal Unbundle", "Terminal Bundle", "Bundler Move Up", "Bundler Move Down", "Bundler Insert", "Bundler Remove", "Bundler Remove Unwired", "Bundler Rearrange", "In Place Insert", "In Place Remove", "In Place Remove Unwired", "In Place Rearrange", "Wire Properties", "Wire Method", "Terminal Properties", "Terminal Method", "Property Move Up", "Property Move Down", "Properties Insert", "Properties Remove", "Properties Remove Unwired", "Properties Rearrange", "Method Change", "Class For Constant", "Class For Control", "Class For Node", "Class Name to Clipboard"}
  T7 = typedef "eventvkey.ctl" = enum16{"ASCII", "Enter", "Return", "Shift", "Ctrl", "Alt", "Cmd", "Opt", "Caps", "NumLock", "Clear", "Break", "Up", "Down", "Left", "Right", "Insert", "Delete", "Home", "End", "PageUp", "PageDown", "Escape", "Help", "Pause", "ScrollLock", "F1", "F2", "F3", "F4", "F5", "F6", "F7", "F8", "F9", "F10", "F11", "F12", "F13", "F14", "F15", "F16", "F17", "F18", "F19", "F20", "F21", "F22", "F23", "F24", "Play", "VolumeUp", "VolumeDown", "Mute", "Two Byte Char"}
  T8 = enum16{"Init", "Read", "Remove", "Remove or Append", "Append", "Append If New"}
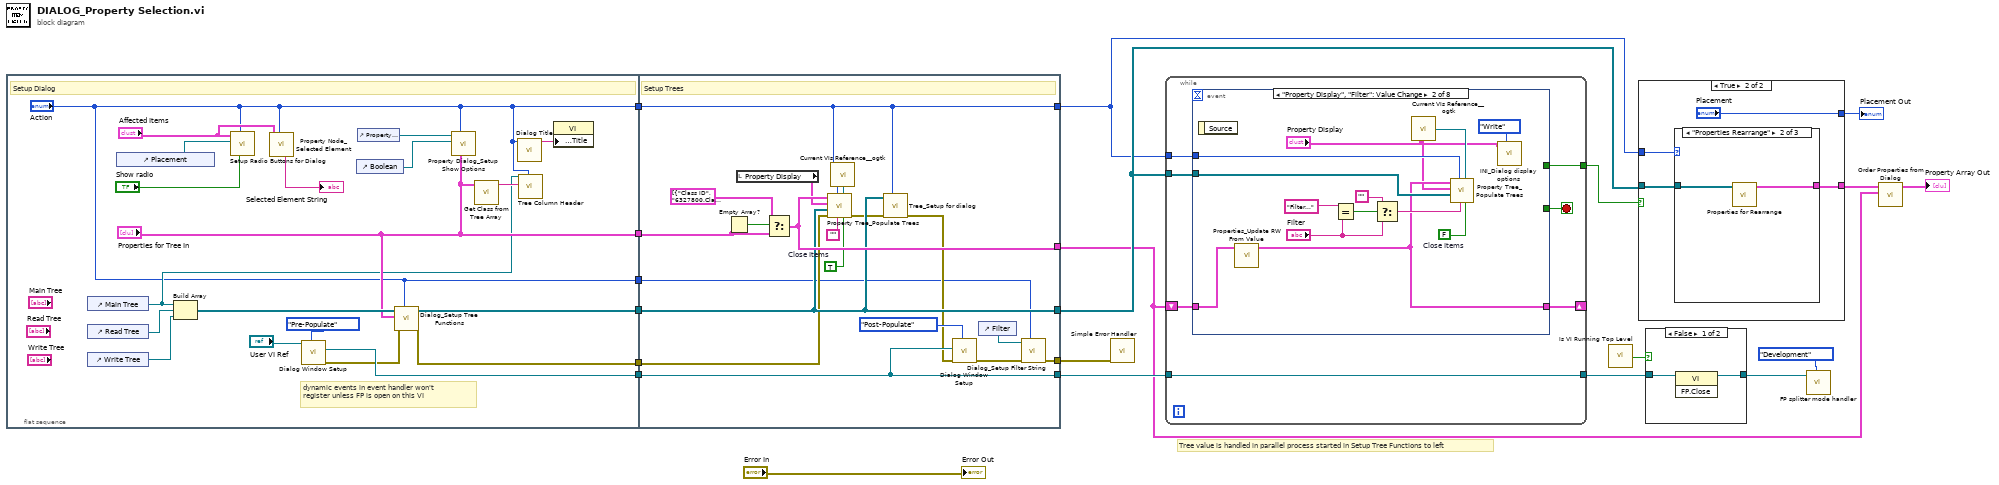
[diagram p0: block diagram]
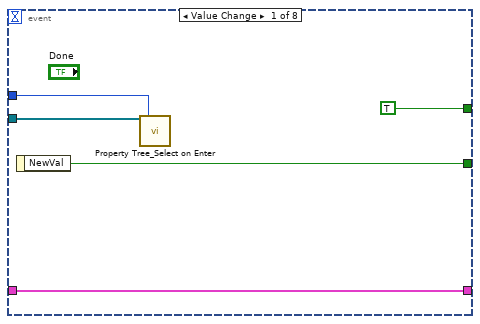
[diagram p2: hidden frame]
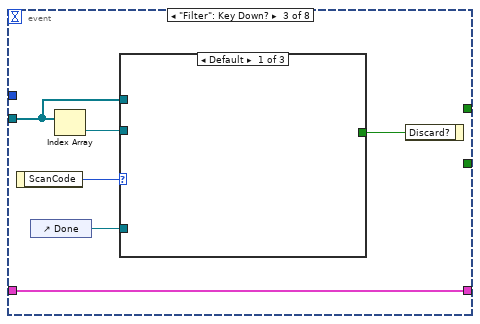
[diagram p3: hidden frame]
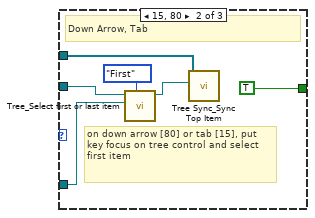
[diagram p4: hidden frame]
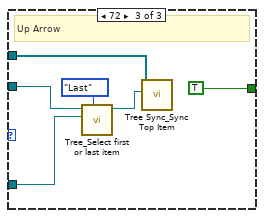
[diagram p5: hidden frame]
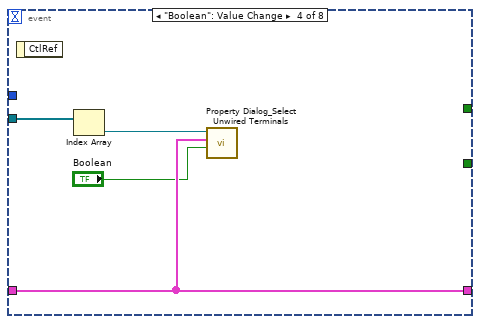
[diagram p6: hidden frame]
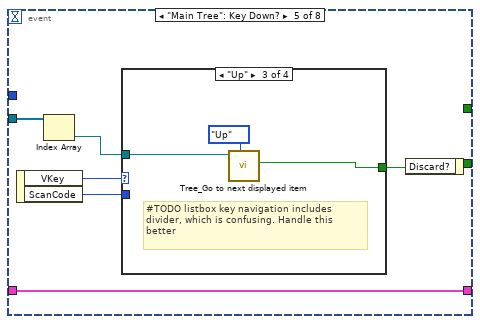
[diagram p7: hidden frame]
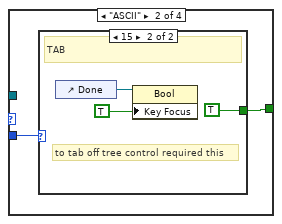
[diagram p9: hidden frame]
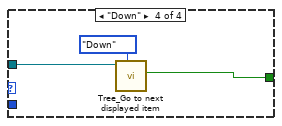
[diagram p11: hidden frame]
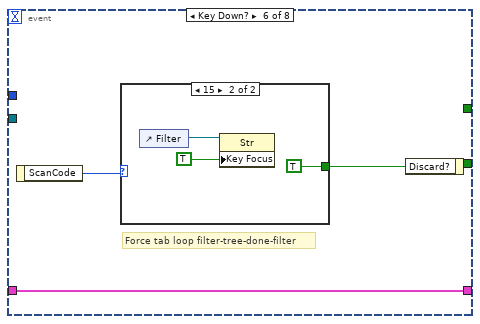
[diagram p12: hidden frame]
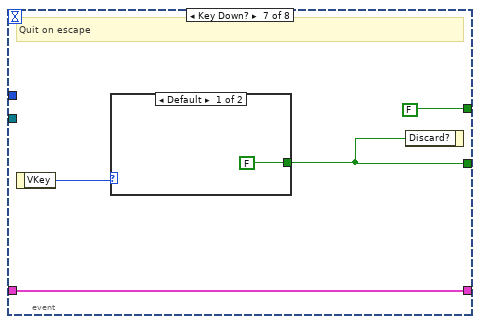
[diagram p14: hidden frame]
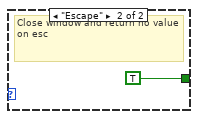
[diagram p15: hidden frame]
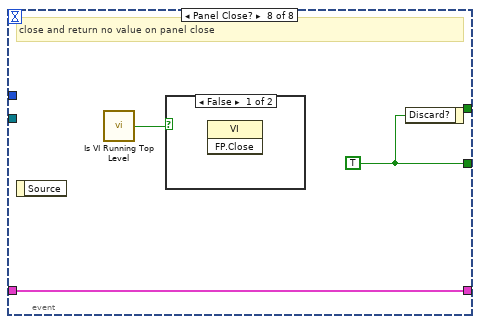
[diagram p16: hidden frame]
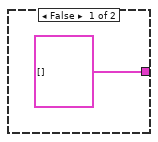
[diagram p19: hidden frame]
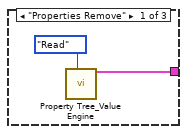
[diagram p20: hidden frame]
diagram:
  # "Tree value is handled in parallel process started in Setup Tree Functions to left"
  n1 = flat-sequence {
    tunnel: [w37] -> w12
    tunnel: [w32] -> w11
    tunnel: ["Action"] -> w10
    tunnel: ["Properties for Tree In"] -> w5
    tunnel: [w22] -> w3
    tunnel: ["Action"] -> w1
    tunnel: [w55] -> w13
    tunnel: [w49] -> w18
    tunnel: w12 -> [w49]
    tunnel: w11 -> [w55]
    tunnel: [w57] -> w6
    tunnel: w10 -> [w56]
    tunnel: [w56] -> w9
    tunnel: w5 -> [w51]
    tunnel: w3 -> [w45]
    tunnel: [w42] -> w2
    tunnel: w1 -> [w41]
    frame #0 {
      # "dynamic events in event handler won't register unless FP is open on this VI"
      # "Setup Dialog"
      n2 = control-ref of="Main Tree"() -> (w23:refnum<vi>)
      n3 = control-ref of="Read Tree"() -> (w36:refnum<vi>)
      n4 = control-ref of="Write Tree"() -> (w35:refnum<vi>)
      n5 = control-ref of="Placement"() -> (w39:refnum<vi>)
      n6 = Build Array(w23, w36, w35) -> (w31:refnum<vi>[])
      n7 = call "Setup Radio Buttons for Dialog.vi"("Show Radio"="Show radio", "Action"="Action", "Action Choice Ref"=w39, "Affected Items"="Affected Items") -> ()  [unwired: 8 in]
      n8 = call "Property Node_Selected Element.vi"("Action"="Action", "Affected Items"="Affected Items") -> ("Display String"=→"Selected Element String":string)  [unwired: 4 in, 5 out]
      n9 = call "Dialog Window Setup.vi"("Action"=enum16{"Pre-Populate", "Post-Populate"}."Pre-Populate", "Align-to Window Ref"="User VI Ref") -> ("error out"=w33:errorcluster, "Dialog VI Ref Out"=w37:refnum<vi>)  [unwired: 8 in]
      n10 = control-ref of="Boolean"() -> (w30:refnum<vi>)
      n11 = control-ref of="Property Display"() -> (w34:refnum<vi>)
      n12 = call "Dialog_Setup Tree Functions.vi"("Action"="Action", "error in"=w33, "Properties for Tree In"="Properties for Tree In", "Tree Ref Array In"=w31) -> ("error out"=w22:errorcluster, "Tree Ref Array Out"=w32:refnum<vi>[])  [unwired: 6 in]
      n13 = call "Property Dialog_Setup Show Options.vi"("Properties for Tree In"="Properties for Tree In", "Action"="Action", "Select Unwired Ref"=w30, "Cluster in"=w34) -> ()  [unwired: 8 in]
      n14 = call "Get Class from Tree Array.vi"("Methods for Tree In"="Properties for Tree In") -> ("Class"=w25:string)  [unwired: 10 in]
      n15 = call "Dialog Title.vi"("Action"="Action") -> ("Window Title"=w29:string)  [unwired: 10 in]
      n16 = call "Tree Column Header.vi"("Action"="Action", "Class Name"=w25, "Tree Ref"=w23) -> ()  [unwired: 8 in, 1 out]
      n17 = property class="VI"("Front Panel.Title"=w29) -> ()  [unwired: 2 in, 2 out]
    }
    frame #1 {
      w50 = TRUE  # Close Items
      # "Setup Trees"
      n18 = Empty Array?(array=w51) -> (empty?=w59:bool)
      n19 = local read "Property Display"() -> (w54:T1)
      n20 = Select(t=T5 [{"Label"="Class ID", "Tag"="6327800.Class ID", "Property Type"=enum."Base", "Indent"=0, "Can Read?"=TRUE, "Can Write?"=FALSE, "Is Read?"=FALSE, "Is Write?"=FALSE, "Inactive Parent?"=FALSE, "Unwired?"=FALSE}, {"Label"="Class Name", "Tag"="6327803.Class Name", "Property Type"=enum."Base", "Indent"=0, "Can Read?"=TRUE, "Can Write?"=FALSE, "Is Read?"=FALSE, "Is Write?"=FALSE, "Inactive Parent?"=FALSE, "Unwired?"=FALSE}, {"Label"="Is On Block Diagram?", "Tag"="6327805.Is On Block Diagram?", "Property Type"=enum."Scripting", "Indent"=0, "Can Read?"=TRUE, "Can Write?"=FALSE, "Is Read?"=FALSE, "Is Write?"=FALSE, "Inactive Parent?"=FALSE, "Unwired?"=FALSE}, {"Label"="Modified", "Tag"="6327804.Modified", "Property Type"=enum."Private", "Indent"=0, "Can Read?"=TRUE, "Can Write?"=FALSE, "Is Read?"=FALSE, "Is Write?"=FALSE, "Inactive Parent?"=FALSE, "Unwired?"=FALSE}, {"Label"="Owner", "Tag"="6327806.Owner", "Property Type"=enum."Base", "Indent"=0, "Can Read?"=TRUE, "Can Write?"=FALSE, "Is Read?"=FALSE, "Is Write?"=FALSE, "Inactive Parent?"=FALSE, "Unwired?"=FALSE}, {"Label"="Owning VI", "Tag"="6327802.Owning VI", "Property Type"=enum."Base", "Indent"=0, "Can Read?"=TRUE, "Can Write?"=FALSE, "Is Read?"=FALSE, "Is Write?"=FALSE, "Inactive Parent?"=FALSE, "Unwired?"=FALSE}, {"Label"="Basic Object Flags", "Tag"="632a80c.Basic Object Flags", "Property Type"=enum."Private", "Indent"=0, "Can Read?"=TRUE, "Can Write?"=TRUE, "Is Read?"=FALSE, "Is Write?"=FALSE, "Inactive Parent?"=FALSE, "Unwired?"=FALSE}, {"Label"="Bounds", "Tag"="632a803.Bounds", "Property Type"=enum."Base", "Indent"=0, "Can Read?"=TRUE, "Can Write?"=FALSE, "Is Read?"=FALSE, "Is Write?"=FALSE, "Inactive Parent?"=FALSE, "Unwired?"=FALSE}, {"Label"="Area Height", "Tag"="632a805.Bounds:Area Height", "Property Type"=enum."Base", "Indent"=1, "Can Read?"=TRUE, "Can Write?"=FALSE, "Is Read?"=FALSE, "Is Write?"=FALSE, "Inactive Parent?"=FALSE, "Unwired?"=FALSE}, {"Label"="Area Width", "Tag"="632a804.Bounds:Area Width", "Property Type"=enum."Base", "Indent"=1, "Can Read?"=TRUE, "Can Write?"=FALSE, "Is Read?"=FALSE, "Is Write?"=FALSE, "Inactive Parent?"=FALSE, "Unwired?"=FALSE}, {"Label"="Dependencies", "Tag"="Dependencies", "Property Type"=enum."Scripting", "Indent"=0, "Can Read?"=FALSE, "Can Write?"=FALSE, "Is Read?"=FALSE, "Is Write?"=FALSE, "Inactive Parent?"=TRUE, "Unwired?"=FALSE}, {"Label"="Found Dependency Names", "Tag"="632a817.Dependencies:Found Dependency Names", "Property Type"=enum."Scripting", "Indent"=1, "Can Read?"=TRUE, "Can Write?"=FALSE, "Is Read?"=FALSE, "Is Write?"=FALSE, "Inactive Parent?"=FALSE, "Unwired?"=FALSE}, {"Label"="Found Dependency Paths", "Tag"="632a816.Dependencies:Found Dependency Paths", "Property Type"=enum."Scripting", "Indent"=1, "Can Read?"=TRUE, "Can Write?"=FALSE, "Is Read?"=FALSE, "Is Write?"=FALSE, "Inactive Parent?"=FALSE, "Unwired?"=FALSE}, {"Label"="Missing Dependency Names", "Tag"="632a815.Dependencies:Missing Dependency Names", "Property Type"=enum."Scripting", "Indent"=1, "Can Read?"=TRUE, "Can Write?"=FALSE, "Is Read?"=FALSE, "Is Write?"=FALSE, "Inactive Parent?"=FALSE, "Unwired?"=FALSE}, {"Label"="Missing Dependency Paths", "Tag"="632a814.Dependencies:Missing Dependency Paths", "Property Type"=enum."Scripting", "Indent"=1, "Can Read?"=TRUE, "Can Write?"=FALSE, "Is Read?"=FALSE, "Is Write?"=FALSE, "Inactive Parent?"=FALSE, "Unwired?"=FALSE}, {"Label"="Group Member Refs[]", "Tag"="632a808.Group Member Refs[]", "Property Type"=enum."Private", "Indent"=0, "Can Read?"=TRUE, "Can Write?"=FALSE, "Is Read?"=FALSE, "Is Write?"=FALSE, "Inactive Parent?"=FALSE, "Unwired?"=FALSE}, {"Label"="Grouped", "Tag"="632a806.Grouped", "Property Type"=enum."Private", "Indent"=0, "Can Read?"=TRUE, "Can Write?"=FALSE, "Is Read?"=FALSE, "Is Write?"=FALSE, "Inactive Parent?"=FALSE, "Unwired?"=FALSE}, {"Label"="Is Wizard Locked", "Tag"="632a80d.Is Wizard Locked", "Property Type"=enum."Private", "Indent"=0, "Can Read?"=TRUE, "Can Write?"=FALSE, "Is Read?"=FALSE, "Is Write?"=FALSE, "Inactive Parent?"=FALSE, "Unwired?"=FALSE}, {"Label"="Locked", "Tag"="632a807.Locked", "Property Type"=enum."Private", "Indent"=0, "Can Read?"=TRUE, "Can Write?"=FALSE, "Is Read?"=FALSE, "Is Write?"=FALSE, "Inactive Parent?"=FALSE, "Unwired?"=FALSE}, {"Label"="Master Bounds Rect", "Tag"="632a80b.Master Bounds Rect", "Property Type"=enum."Scripting", "Indent"=0, "Can Read?"=TRUE, "Can Write?"=FALSE, "Is Read?"=FALSE, "Is Write?"=FALSE, "Inactive Parent?"=FALSE, "Unwired?"=FALSE}, {"Label"="Position", "Tag"="632a800.Position", "Property Type"=enum."Base", "Indent"=0, "Can Read?"=TRUE, "Can Write?"=TRUE, "Is Read?"=FALSE, "Is Write?"=FALSE, "Inactive Parent?"=FALSE, "Unwired?"=FALSE}, {"Label"="Left", "Tag"="632a801.Position:Left", "Property Type"=enum."Base", "Indent"=1, "Can Read?"=TRUE, "Can Write?"=TRUE, "Is Read?"=FALSE, "Is Write?"=FALSE, "Inactive Parent?"=FALSE, "Unwired?"=FALSE}, {"Label"="Top", "Tag"="632a802.Position:Top", "Property Type"=enum."Base", "Indent"=1, "Can Read?"=TRUE, "Can Write?"=TRUE, "Is Read?"=FALSE, "Is Write?"=FALSE, "Inactive Parent?"=FALSE, "Unwired?"=FALSE}, {"Label"="Resize Info", "Tag"="Resize Info", "Property Type"=enum."Private", "Indent"=0, "Can Read?"=FALSE, "Can Write?"=FALSE, "Is Read?"=FALSE, "Is Write?"=FALSE, "Inactive Parent?"=TRUE, "Unwired?"=FALSE}, {"Label"="Can Resize Horizontally", "Tag"="632a80f.Resize Info:Can Resize Horizontally", "Property Type"=enum."Private", "Indent"=1, "Can Read?"=TRUE, "Can Write?"=FALSE, "Is Read?"=FALSE, "Is Write?"=FALSE, "Inactive Parent?"=FALSE, "Unwired?"=FALSE}, {"Label"="Can Resize Vertically", "Tag"="632a810.Resize Info:Can Resize Vertically", "Property Type"=enum."Private", "Indent"=1, "Can Read?"=TRUE, "Can Write?"=FALSE, "Is Read?"=FALSE, "Is Write?"=FALSE, "Inactive Parent?"=FALSE, "Unwired?"=FALSE}, {"Label"="Include In Resize", "Tag"="632a812.Resize Info:Include In Resize", "Property Type"=enum."Private", "Indent"=1, "Can Read?"=TRUE, "Can Write?"=FALSE, "Is Read?"=FALSE, "Is Write?"=FALSE, "Inactive Parent?"=FALSE, "Unwired?"=FALSE}, {"Label"="Name in Resize Dialog", "Tag"="632a811.Resize Info:Name in Resize Dialog", "Property Type"=enum."Private", "Indent"=1, "Can Read?"=TRUE, "Can Write?"=FALSE, "Is Read?"=FALSE, "Is Write?"=FALSE, "Inactive Parent?"=FALSE, "Unwired?"=FALSE}, {"Label"="Selected", "Tag"="632a809.Selected", "Property Type"=enum."Scripting", "Indent"=0, "Can Read?"=TRUE, "Can Write?"=TRUE, "Is Read?"=FALSE, "Is Write?"=FALSE, "Inactive Parent?"=FALSE, "Unwired?"=FALSE}, {"Label"="Total Bounds Rect", "Tag"="632a80a.Total Bounds Rect", "Property Type"=enum."Scripting", "Indent"=0, "Can Read?"=TRUE, "Can Write?"=FALSE, "Is Read?"=FALSE, "Is Write?"=FALSE, "Inactive Parent?"=FALSE, "Unwired?"=FALSE}, {"Label"="UID", "Tag"="632a813.UID", "Property Type"=enum."Scripting", "Indent"=0, "Can Read?"=TRUE, "Can Write?"=FALSE, "Is Read?"=FALSE, "Is Write?"=FALSE, "Inactive Parent?"=FALSE, "Unwired?"=FALSE}, {"Label"="Auto-Update From Typedef", "Tag"="633201c.Auto-Update From Typedef", "Property Type"=enum."Scripting", "Indent"=0, "Can Read?"=TRUE, "Can Write?"=TRUE, "Is Read?"=FALSE, "Is Write?"=FALSE, "Inactive Parent?"=FALSE, "Unwired?"=FALSE}, {"Label"="Bit Accurate Data Size", "Tag"="633201d.Bit Accurate Data Size", "Property Type"=enum."Private", "Indent"=0, "Can Read?"=TRUE, "Can Write?"=FALSE, "Is Read?"=FALSE, "Is Write?"=FALSE, "Inactive Parent?"=FALSE, "Unwired?"=FALSE}, {"Label"="Blinking", "Tag"="6332003.Blinking", "Property Type"=enum."Base", "Indent"=0, "Can Read?"=TRUE, "Can Write?"=TRUE, "Is Read?"=FALSE, "Is Write?"=FALSE, "Inactive Parent?"=FALSE, "Unwired?"=FALSE}, {"Label"="Built-In Mouse Wheel Support", "Tag"="633203f.Built-In Mouse Wheel Support", "Property Type"=enum."Base", "Indent"=0, "Can Read?"=TRUE, "Can Write?"=TRUE, "Is Read?"=FALSE, "Is Write?"=FALSE, "Inactive Parent?"=FALSE, "Unwired?"=FALSE}, {"Label"="C Type", "Tag"="6332026.C Type", "Property Type"=enum."Private", "Indent"=0, "Can Read?"=TRUE, "Can Write?"=FALSE, "Is Read?"=FALSE, "Is Write?"=FALSE, "Inactive Parent?"=FALSE, "Unwired?"=FALSE}, {"Label"="Caption", "Tag"="6332004.Caption", "Property Type"=enum."Base", "Indent"=0, "Can Read?"=TRUE, "Can Write?"=FALSE, "Is Read?"=FALSE, "Is Write?"=FALSE, "Inactive Parent?"=FALSE, "Unwired?"=FALSE}, {"Label"="Control Index", "Tag"="6332040.Control Index", "Property Type"=enum."Base", "Indent"=0, "Can Read?"=TRUE, "Can Write?"=FALSE, "Is Read?"=FALSE, "Is Write?"=FALSE, "Inactive Parent?"=FALSE, "Unwired?"=FALSE}, {"Label"="Control Reference Nodes[]", "Tag"="6332009.Control Reference Nodes[]", "Property Type"=enum."Scripting", "Indent"=0, "Can Read?"=TRUE, "Can Write?"=FALSE, "Is Read?"=FALSE, "Is Write?"=FALSE, "Inactive Parent?"=FALSE, "Unwired?"=FALSE}, {"Label"="Data Binding", "Tag"="Data Binding", "Property Type"=enum."Base", "Indent"=0, "Can Read?"=FALSE, "Can Write?"=FALSE, "Is Read?"=FALSE, "Is Write?"=FALSE, "Inactive Parent?"=TRUE, "Unwired?"=FALSE}, {"Label"="Binding Type", "Tag"="633202d.Data Binding:Binding Type", "Property Type"=enum."Base", "Indent"=1, "Can Read?"=TRUE, "Can Write?"=FALSE, "Is Read?"=FALSE, "Is Write?"=FALSE, "Inactive Parent?"=FALSE, "Unwired?"=FALSE}, {"Label"="Blink On Alarm", "Tag"="633202e.Data Binding:Blink On Alarm", "Property Type"=enum."Private", "Indent"=1, "Can Read?"=TRUE, "Can Write?"=TRUE, "Is Read?"=FALSE, "Is Write?"=FALSE, "Inactive Parent?"=FALSE, "Unwired?"=FALSE}, {"Label"="LED Visible", "Tag"="633202b.Data Binding:LED Visible", "Property Type"=enum."Base", "Indent"=1, "Can Read?"=TRUE, "Can Write?"=TRUE, "Is Read?"=FALSE, "Is Write?"=FALSE, "Inactive Parent?"=FALSE, "Unwired?"=FALSE}, {"Label"="Mode", "Tag"="6332029.Data Binding:Mode", "Property Type"=enum."Base", "Indent"=1, "Can Read?"=TRUE, "Can Write?"=TRUE, "Is Read?"=FALSE, "Is Write?"=FALSE, "Inactive Parent?"=FALSE, "Unwired?"=FALSE}, {"Label"="Path", "Tag"="6332028.Data Binding:Path", "Property Type"=enum."Base", "Indent"=1, "Can Read?"=TRUE, "Can Write?"=TRUE, "Is Read?"=FALSE, "Is Write?"=FALSE, "Inactive Parent?"=FALSE, "Unwired?"=FALSE}, {"Label"="Persist ID", "Tag"="633202c.Data Binding:Persist ID", "Property Type"=enum."Private", "Indent"=1, "Can Read?"=TRUE, "Can Write?"=FALSE, "Is Read?"=FALSE, "Is Write?"=FALSE, "Inactive Parent?"=FALSE, "Unwired?"=FALSE}, {"Label"="Status", "Tag"="633202a.Data Binding:Status", "Property Type"=enum."Base", "Indent"=1, "Can Read?"=TRUE, "Can Write?"=FALSE, "Is Read?"=FALSE, "Is Write?"=FALSE, "Inactive Parent?"=FALSE, "Unwired?"=FALSE}, {"Label"="DataSocket", "Tag"="DataSocket", "Property Type"=enum."Base", "Indent"=0, "Can Read?"=FALSE, "Can Write?"=FALSE, "Is Read?"=FALSE, "Is Write?"=FALSE, "Inactive Parent?"=TRUE, "Unwired?"=FALSE}, {"Label"="Enabled", "Tag"="6332017.DataSocket:Enabled", "Property Type"=enum."Base", "Indent"=1, "Can Read?"=TRUE, "Can Write?"=TRUE, "Is Read?"=FALSE, "Is Write?"=FALSE, "Inactive Parent?"=FALSE, "Unwired?"=FALSE}, {"Label"="LED Visible", "Tag"="633201e.DataSocket:LED Visible", "Property Type"=enum."Base", "Indent"=1, "Can Read?"=TRUE, "Can Write?"=TRUE, "Is Read?"=FALSE, "Is Write?"=FALSE, "Inactive Parent?"=FALSE, "Unwired?"=FALSE}, {"Label"="Mode", "Tag"="6332016.DataSocket:Mode", "Property Type"=enum."Base", "Indent"=1, "Can Read?"=TRUE, "Can Write?"=TRUE, "Is Read?"=FALSE, "Is Write?"=FALSE, "Inactive Parent?"=FALSE, "Unwired?"=FALSE}, {"Label"="Status", "Tag"="6332018.DataSocket:Status", "Property Type"=enum."Base", "Indent"=1, "Can Read?"=TRUE, "Can Write?"=FALSE, "Is Read?"=FALSE, "Is Write?"=FALSE, "Inactive Parent?"=FALSE, "Unwired?"=FALSE}, {"Label"="URL", "Tag"="6332015.DataSocket:URL", "Property Type"=enum."Base", "Indent"=1, "Can Read?"=TRUE, "Can Write?"=TRUE, "Is Read?"=FALSE, "Is Write?"=FALSE, "Inactive Parent?"=FALSE, "Unwired?"=FALSE}, {"Label"="", "Tag"="", "Property Type"=enum."Base", "Indent"=0, "Can Read?"=FALSE, "Can Write?"=FALSE, "Is Read?"=FALSE, "Is Write?"=FALSE, "Inactive Parent?"=FALSE, "Unwired?"=FALSE}, {"Label"="Default Value (Undoable)", "Tag"="6332043.Default Value (Undoable)", "Property Type"=enum."Scripting", "Indent"=0, "Can Read?"=FALSE, "Can Write?"=TRUE, "Is Read?"=FALSE, "Is Write?"=FALSE, "Inactive Parent?"=FALSE, "Unwired?"=FALSE}, {"Label"="Description", "Tag"="633200f.Description", "Property Type"=enum."Base", "Indent"=0, "Can Read?"=TRUE, "Can Write?"=TRUE, "Is Read?"=FALSE, "Is Write?"=FALSE, "Inactive Parent?"=FALSE, "Unwired?"=FALSE}, {"Label"="Disabled", "Tag"="633203d.Disabled", "Property Type"=enum."Base", "Indent"=0, "Can Read?"=TRUE, "Can Write?"=TRUE, "Is Read?"=FALSE, "Is Write?"=FALSE, "Inactive Parent?"=FALSE, "Unwired?"=FALSE}, {"Label"="Focus Key Binding", "Tag"="6332010.Focus Key Binding", "Property Type"=enum."Base", "Indent"=0, "Can Read?"=TRUE, "Can Write?"=TRUE, "Is Read?"=FALSE, "Is Write?"=FALSE, "Inactive Parent?"=FALSE, "Unwired?"=FALSE}, {"Label"="Genericity", "Tag"="633203c.Genericity", "Property Type"=enum."Private", "Indent"=0, "Can Read?"=TRUE, "Can Write?"=TRUE, "Is Read?"=FALSE, "Is Write?"=FALSE, "Inactive Parent?"=FALSE, "Unwired?"=FALSE}, {"Label"="Grow Info", "Tag"="633202f.Grow Info", "Property Type"=enum."Scripting", "Indent"=0, "Can Read?"=TRUE, "Can Write?"=FALSE, "Is Read?"=FALSE, "Is Write?"=FALSE, "Inactive Parent?"=FALSE, "Unwired?"=FALSE}, {"Label"="Can Grow Horizontally", "Tag"="6332030.Grow Info:Can Grow Horizontally", "Property Type"=enum."Scripting", "Indent"=1, "Can Read?"=TRUE, "Can Write?"=FALSE, "Is Read?"=FALSE, "Is Write?"=FALSE, "Inactive Parent?"=FALSE, "Unwired?"=FALSE}, {"Label"="Can Grow Vertically", "Tag"="6332031.Grow Info:Can Grow Vertically", "Property Type"=enum."Scripting", "Indent"=1, "Can Read?"=TRUE, "Can Write?"=FALSE, "Is Read?"=FALSE, "Is Write?"=FALSE, "Inactive Parent?"=FALSE, "Unwired?"=FALSE}, {"Label"="Max Horizontally", "Tag"="6332034.Grow Info:Max Horizontally", "Property Type"=enum."Scripting", "Indent"=1, "Can Read?"=TRUE, "Can Write?"=FALSE, "Is Read?"=FALSE, "Is Write?"=FALSE, "Inactive Parent?"=FALSE, "Unwired?"=FALSE}, {"Label"="Max Vertically", "Tag"="6332035.Grow Info:Max Vertically", "Property Type"=enum."Scripting", "Indent"=1, "Can Read?"=TRUE, "Can Write?"=FALSE, "Is Read?"=FALSE, "Is Write?"=FALSE, "Inactive Parent?"=FALSE, "Unwired?"=FALSE}, {"Label"="Min Horizontally", "Tag"="6332032.Grow Info:Min Horizontally", "Property Type"=enum."Scripting", "Indent"=1, "Can Read?"=TRUE, "Can Write?"=FALSE, "Is Read?"=FALSE, "Is Write?"=FALSE, "Inactive Parent?"=FALSE, "Unwired?"=FALSE}, {"Label"="Min Vertically", "Tag"="6332033.Grow Info:Min Vertically", "Property Type"=enum."Scripting", "Indent"=1, "Can Read?"=TRUE, "Can Write?"=FALSE, "Is Read?"=FALSE, "Is Write?"=FALSE, "Inactive Parent?"=FALSE, "Unwired?"=FALSE}, {"Label"="Has Caption", "Tag"="6332022.Has Caption", "Property Type"=enum."Scripting", "Indent"=0, "Can Read?"=TRUE, "Can Write?"=FALSE, "Is Read?"=FALSE, "Is Write?"=FALSE, "Inactive Parent?"=FALSE, "Unwired?"=FALSE}, {"Label"="Indicator", "Tag"="6332007.Indicator", "Property Type"=enum."Base", "Indent"=0, "Can Read?"=TRUE, "Can Write?"=TRUE, "Is Read?"=FALSE, "Is Write?"=FALSE, "Inactive Parent?"=FALSE, "Unwired?"=FALSE}, {"Label"="Invoke Nodes[]", "Tag"="633200c.Invoke Nodes[]", "Property Type"=enum."Scripting", "Indent"=0, "Can Read?"=TRUE, "Can Write?"=FALSE, "Is Read?"=FALSE, "Is Write?"=FALSE, "Inactive Parent?"=FALSE, "Unwired?"=FALSE}, {"Label"="Is On Connector Pane", "Tag"="6332020.Is On Connector Pane", "Property Type"=enum."Scripting", "Indent"=0, "Can Read?"=TRUE, "Can Write?"=FALSE, "Is Read?"=FALSE, "Is Write?"=FALSE, "Inactive Parent?"=FALSE, "Unwired?"=FALSE}, {"Label"="Is Stub?", "Tag"="633203b.Is Stub?", "Property Type"=enum."Private", "Indent"=0, "Can Read?"=TRUE, "Can Write?"=FALSE, "Is Read?"=FALSE, "Is Write?"=FALSE, "Inactive Parent?"=FALSE, "Unwired?"=FALSE}, {"Label"="Is Typedef?", "Tag"="633201a.Is Typedef?", "Property Type"=enum."Scripting", "Indent"=0, "Can Read?"=TRUE, "Can Write?"=FALSE, "Is Read?"=FALSE, "Is Write?"=FALSE, "Inactive Parent?"=FALSE, "Unwired?"=FALSE}, {"Label"="Key Focus", "Tag"="6332002.Key Focus", "Property Type"=enum."Base", "Indent"=0, "Can Read?"=TRUE, "Can Write?"=TRUE, "Is Read?"=FALSE, "Is Write?"=FALSE, "Inactive Parent?"=FALSE, "Unwired?"=FALSE}, {"Label"="Label", "Tag"="6332005.Label", "Property Type"=enum."Base", "Indent"=0, "Can Read?"=TRUE, "Can Write?"=FALSE, "Is Read?"=FALSE, "Is Write?"=FALSE, "Inactive Parent?"=FALSE, "Unwired?"=FALSE}, {"Label"="Latch Value", "Tag"="633201f.Latch Value", "Property Type"=enum."Private", "Indent"=0, "Can Read?"=TRUE, "Can Write?"=TRUE, "Is Read?"=FALSE, "Is Write?"=FALSE, "Inactive Parent?"=FALSE, "Unwired?"=FALSE}, {"Label"="Local Variables[]", "Tag"="633200a.Local Variables[]", "Property Type"=enum."Scripting", "Indent"=0, "Can Read?"=TRUE, "Can Write?"=FALSE, "Is Read?"=FALSE, "Is Write?"=FALSE, "Inactive Parent?"=FALSE, "Unwired?"=FALSE}, {"Label"="Owning Pane", "Tag"="633203e.Owning Pane", "Property Type"=enum."Base", "Indent"=0, "Can Read?"=TRUE, "Can Write?"=FALSE, "Is Read?"=FALSE, "Is Write?"=FALSE, "Inactive Parent?"=FALSE, "Unwired?"=FALSE}, {"Label"="Property Nodes[]", "Tag"="633200b.Property Nodes[]", "Property Type"=enum."Scripting", "Indent"=0, "Can Read?"=TRUE, "Can Write?"=FALSE, "Is Read?"=FALSE, "Is Write?"=FALSE, "Inactive Parent?"=FALSE, "Unwired?"=FALSE}, {"Label"="Skip When Tabbing", "Tag"="6332021.Skip When Tabbing", "Property Type"=enum."Base", "Indent"=0, "Can Read?"=TRUE, "Can Write?"=TRUE, "Is Read?"=FALSE, "Is Write?"=FALSE, "Inactive Parent?"=FALSE, "Unwired?"=FALSE}, {"Label"="Style ID", "Tag"="633203a.Style ID", "Property Type"=enum."Scripting", "Indent"=0, "Can Read?"=TRUE, "Can Write?"=FALSE, "Is Read?"=FALSE, "Is Write?"=FALSE, "Inactive Parent?"=FALSE, "Unwired?"=FALSE}, {"Label"="Synchronous Display", "Tag"="6332008.Synchronous Display", "Property Type"=enum."Base", "Indent"=0, "Can Read?"=TRUE, "Can Write?"=TRUE, "Is Read?"=FALSE, "Is Write?"=FALSE, "Inactive Parent?"=FALSE, "Unwired?"=FALSE}, {"Label"="Terminal", "Tag"="6332006.Terminal", "Property Type"=enum."Scripting", "Indent"=0, "Can Read?"=TRUE, "Can Write?"=FALSE, "Is Read?"=FALSE, "Is Write?"=FALSE, "Inactive Parent?"=FALSE, "Unwired?"=FALSE}, {"Label"="Tip Strip", "Tag"="6332014.Tip Strip", "Property Type"=enum."Base", "Indent"=0, "Can Read?"=TRUE, "Can Write?"=TRUE, "Is Read?"=FALSE, "Is Write?"=FALSE, "Inactive Parent?"=FALSE, "Unwired?"=FALSE}, {"Label"="Typedef", "Tag"="Typedef", "Property Type"=enum."Scripting", "Indent"=0, "Can Read?"=FALSE, "Can Write?"=FALSE, "Is Read?"=FALSE, "Is Write?"=FALSE, "Inactive Parent?"=TRUE, "Unwired?"=FALSE}, {"Label"="Path", "Tag"="633201b.Typedef:Path", "Property Type"=enum."Scripting", "Indent"=1, "Can Read?"=TRUE, "Can Write?"=FALSE, "Is Read?"=FALSE, "Is Write?"=FALSE, "Inactive Parent?"=FALSE, "Unwired?"=FALSE}, {"Label"="VI", "Tag"="6332025.Typedef:VI", "Property Type"=enum."Scripting", "Indent"=1, "Can Read?"=TRUE, "Can Write?"=FALSE, "Is Read?"=FALSE, "Is Write?"=FALSE, "Inactive Parent?"=FALSE, "Unwired?"=FALSE}, {"Label"="", "Tag"="", "Property Type"=enum."Base", "Indent"=0, "Can Read?"=FALSE, "Can Write?"=FALSE, "Is Read?"=FALSE, "Is Write?"=FALSE, "Inactive Parent?"=FALSE, "Unwired?"=FALSE}, {"Label"="", "Tag"="", "Property Type"=enum."Base", "Indent"=0, "Can Read?"=FALSE, "Can Write?"=FALSE, "Is Read?"=FALSE, "Is Write?"=FALSE, "Inactive Parent?"=FALSE, "Unwired?"=FALSE}, {"Label"="Value (Undoable)", "Tag"="6332041.Value (Undoable)", "Property Type"=enum."Scripting", "Indent"=0, "Can Read?"=FALSE, "Can Write?"=TRUE, "Is Read?"=FALSE, "Is Write?"=FALSE, "Inactive Parent?"=FALSE, "Unwired?"=FALSE}, {"Label"="Visible", "Tag"="6332000.Visible", "Property Type"=enum."Base", "Indent"=0, "Can Read?"=TRUE, "Can Write?"=TRUE, "Is Read?"=FALSE, "Is Write?"=FALSE, "Inactive Parent?"=FALSE, "Unwired?"=FALSE}, {"Label"="Wizard Data", "Tag"="6332019.Wizard Data", "Property Type"=enum."Private", "Indent"=0, "Can Read?"=TRUE, "Can Write?"=TRUE, "Is Read?"=FALSE, "Is Write?"=FALSE, "Inactive Parent?"=FALSE, "Unwired?"=FALSE}, {"Label"="XControl", "Tag"="XControl", "Property Type"=enum."Base", "Indent"=0, "Can Read?"=FALSE, "Can Write?"=FALSE, "Is Read?"=FALSE, "Is Write?"=FALSE, "Inactive Parent?"=TRUE, "Unwired?"=FALSE}, {"Label"="Container Bounds", "Tag"="6332037.XControl:Container Bounds", "Property Type"=enum."Base", "Indent"=1, "Can Read?"=TRUE, "Can Write?"=TRUE, "Is Read?"=FALSE, "Is Write?"=FALSE, "Inactive Parent?"=FALSE, "Unwired?"=FALSE}, {"Label"="XControl", "Tag"="XControl", "Property Type"=enum."Base", "Indent"=1, "Can Read?"=FALSE, "Can Write?"=FALSE, "Is Read?"=FALSE, "Is Write?"=FALSE, "Inactive Parent?"=TRUE, "Unwired?"=FALSE}, {"Label"="Container Bounds:Height", "Tag"="6332039.XControl:Container Bounds:Height", "Property Type"=enum."Base", "Indent"=2, "Can Read?"=TRUE, "Can Write?"=TRUE, "Is Read?"=FALSE, "Is Write?"=FALSE, "Inactive Parent?"=FALSE, "Unwired?"=FALSE}, {"Label"="Container Bounds:Width", "Tag"="6332038.XControl:Container Bounds:Width", "Property Type"=enum."Base", "Indent"=2, "Can Read?"=TRUE, "Can Write?"=TRUE, "Is Read?"=FALSE, "Is Write?"=FALSE, "Inactive Parent?"=FALSE, "Unwired?"=FALSE}, {"Label"="XControl", "Tag"="XControl", "Property Type"=enum."Base", "Indent"=0, "Can Read?"=FALSE, "Can Write?"=FALSE, "Is Read?"=FALSE, "Is Write?"=FALSE, "Inactive Parent?"=TRUE, "Unwired?"=FALSE}, {"Label"="Is XControl?", "Tag"="6332036.XControl:Is XControl?", "Property Type"=enum."Base", "Indent"=1, "Can Read?"=TRUE, "Can Write?"=FALSE, "Is Read?"=FALSE, "Is Write?"=FALSE, "Inactive Parent?"=FALSE, "Unwired?"=FALSE}, {"Label"="Adapt To Source", "Tag"="633b01e.Adapt To Source", "Property Type"=enum."Scripting", "Indent"=0, "Can Read?"=TRUE, "Can Write?"=TRUE, "Is Read?"=FALSE, "Is Write?"=FALSE, "Inactive Parent?"=FALSE, "Unwired?"=FALSE}, {"Label"="Data Entry Limits", "Tag"="633b004.Data Entry Limits", "Property Type"=enum."Base", "Indent"=0, "Can Read?"=TRUE, "Can Write?"=TRUE, "Is Read?"=FALSE, "Is Write?"=FALSE, "Inactive Parent?"=FALSE, "Unwired?"=FALSE}, {"Label"="Increment", "Tag"="633b007.Data Entry Limits:Increment", "Property Type"=enum."Base", "Indent"=1, "Can Read?"=TRUE, "Can Write?"=TRUE, "Is Read?"=FALSE, "Is Write?"=FALSE, "Inactive Parent?"=FALSE, "Unwired?"=FALSE}, {"Label"="Maximum", "Tag"="633b006.Data Entry Limits:Maximum", "Property Type"=enum."Base", "Indent"=1, "Can Read?"=TRUE, "Can Write?"=TRUE, "Is Read?"=FALSE, "Is Write?"=FALSE, "Inactive Parent?"=FALSE, "Unwired?"=FALSE}, {"Label"="Minimum", "Tag"="633b005.Data Entry Limits:Minimum", "Property Type"=enum."Base", "Indent"=1, "Can Read?"=TRUE, "Can Write?"=TRUE, "Is Read?"=FALSE, "Is Write?"=FALSE, "Inactive Parent?"=FALSE, "Unwired?"=FALSE}, {"Label"="Decrement Key Binding", "Tag"="633b011.Decrement Key Binding", "Property Type"=enum."Base", "Indent"=0, "Can Read?"=TRUE, "Can Write?"=TRUE, "Is Read?"=FALSE, "Is Write?"=FALSE, "Inactive Parent?"=FALSE, "Unwired?"=FALSE}, {"Label"="Fixed-Point Overflow Status Visible?", "Tag"="633b020.Fixed-Point Overflow Status Visible?", "Property Type"=enum."Private", "Indent"=0, "Can Read?"=TRUE, "Can Write?"=TRUE, "Is Read?"=FALSE, "Is Write?"=FALSE, "Inactive Parent?"=FALSE, "Unwired?"=FALSE}, {"Label"="Fixed-Point Representation", "Tag"="Fixed-Point Representation", "Property Type"=enum."Private", "Indent"=0, "Can Read?"=FALSE, "Can Write?"=FALSE, "Is Read?"=FALSE, "Is Write?"=FALSE, "Inactive Parent?"=TRUE, "Unwired?"=FALSE}, {"Label"="Actual", "Tag"="633b01a.Fixed-Point Representation:Actual", "Property Type"=enum."Private", "Indent"=1, "Can Read?"=TRUE, "Can Write?"=FALSE, "Is Read?"=FALSE, "Is Write?"=FALSE, "Inactive Parent?"=FALSE, "Unwired?"=FALSE}, {"Label"="Fixed-Point Representation", "Tag"="Fixed-Point Representation", "Property Type"=enum."Private", "Indent"=1, "Can Read?"=FALSE, "Can Write?"=FALSE, "Is Read?"=FALSE, "Is Write?"=FALSE, "Inactive Parent?"=TRUE, "Unwired?"=FALSE}, {"Label"="Actual:Delta", "Tag"="633b01d.Fixed-Point Representation:Actual:Delta", "Property Type"=enum."Private", "Indent"=2, "Can Read?"=TRUE, "Can Write?"=FALSE, "Is Read?"=FALSE, "Is Write?"=FALSE, "Inactive Parent?"=FALSE, "Unwired?"=FALSE}, {"Label"="Actual:Range Max", "Tag"="633b01c.Fixed-Point Representation:Actual:Range Max", "Property Type"=enum."Private", "Indent"=2, "Can Read?"=TRUE, "Can Write?"=FALSE, "Is Read?"=FALSE, "Is Write?"=FALSE, "Inactive Parent?"=FALSE, "Unwired?"=FALSE}, {"Label"="Actual:Range Min", "Tag"="633b01b.Fixed-Point Representation:Actual:Range Min", "Property Type"=enum."Private", "Indent"=2, "Can Read?"=TRUE, "Can Write?"=FALSE, "Is Read?"=FALSE, "Is Write?"=FALSE, "Inactive Parent?"=FALSE, "Unwired?"=FALSE}, {"Label"="Fixed-Point Representation", "Tag"="Fixed-Point Representation", "Property Type"=enum."Private", "Indent"=0, "Can Read?"=FALSE, "Can Write?"=FALSE, "Is Read?"=FALSE, "Is Write?"=FALSE, "Inactive Parent?"=TRUE, "Unwired?"=FALSE}, {"Label"="Bits", "Tag"="633b012.Fixed-Point Representation:Bits", "Property Type"=enum."Private", "Indent"=1, "Can Read?"=TRUE, "Can Write?"=TRUE, "Is Read?"=FALSE, "Is Write?"=FALSE, "Inactive Parent?"=FALSE, "Unwired?"=FALSE}, {"Label"="Fixed-Point Representation", "Tag"="Fixed-Point Representation", "Property Type"=enum."Private", "Indent"=1, "Can Read?"=FALSE, "Can Write?"=FALSE, "Is Read?"=FALSE, "Is Write?"=FALSE, "Inactive Parent?"=TRUE, "Unwired?"=FALSE}, {"Label"="Bits:Integer Word Length", "Tag"="633b015.Fixed-Point Representation:Bits:Integer Word Length", "Property Type"=enum."Private", "Indent"=2, "Can Read?"=TRUE, "Can Write?"=TRUE, "Is Read?"=FALSE, "Is Write?"=FALSE, "Inactive Parent?"=FALSE, "Unwired?"=FALSE}, {"Label"="Bits:Signed", "Tag"="633b013.Fixed-Point Representation:Bits:Signed", "Property Type"=enum."Private", "Indent"=2, "Can Read?"=TRUE, "Can Write?"=TRUE, "Is Read?"=FALSE, "Is Write?"=FALSE, "Inactive Parent?"=FALSE, "Unwired?"=FALSE}, {"Label"="Bits:Word Length", "Tag"="633b014.Fixed-Point Representation:Bits:Word Length", "Property Type"=enum."Private", "Indent"=2, "Can Read?"=TRUE, "Can Write?"=TRUE, "Is Read?"=FALSE, "Is Write?"=FALSE, "Inactive Parent?"=FALSE, "Unwired?"=FALSE}, {"Label"="Fixed-Point Representation", "Tag"="Fixed-Point Representation", "Property Type"=enum."Private", "Indent"=0, "Can Read?"=FALSE, "Can Write?"=FALSE, "Is Read?"=FALSE, "Is Write?"=FALSE, "Inactive Parent?"=TRUE, "Unwired?"=FALSE}, {"Label"="Desired", "Tag"="633b016.Fixed-Point Representation:Desired", "Property Type"=enum."Private", "Indent"=1, "Can Read?"=TRUE, "Can Write?"=TRUE, "Is Read?"=FALSE, "Is Write?"=FALSE, "Inactive Parent?"=FALSE, "Unwired?"=FALSE}, {"Label"="Fixed-Point Representation", "Tag"="Fixed-Point Representation", "Property Type"=enum."Private", "Indent"=1, "Can Read?"=FALSE, "Can Write?"=FALSE, "Is Read?"=FALSE, "Is Write?"=FALSE, "Inactive Parent?"=TRUE, "Unwired?"=FALSE}, {"Label"="Desired:Delta", "Tag"="633b019.Fixed-Point Representation:Desired:Delta", "Property Type"=enum."Private", "Indent"=2, "Can Read?"=TRUE, "Can Write?"=TRUE, "Is Read?"=FALSE, "Is Write?"=FALSE, "Inactive Parent?"=FALSE, "Unwired?"=FALSE}, {"Label"="Desired:Range Max", "Tag"="633b018.Fixed-Point Representation:Desired:Range Max", "Property Type"=enum."Private", "Indent"=2, "Can Read?"=TRUE, "Can Write?"=TRUE, "Is Read?"=FALSE, "Is Write?"=FALSE, "Inactive Parent?"=FALSE, "Unwired?"=FALSE}, {"Label"="Desired:Range Min", "Tag"="633b017.Fixed-Point Representation:Desired:Range Min", "Property Type"=enum."Private", "Indent"=2, "Can Read?"=TRUE, "Can Write?"=TRUE, "Is Read?"=FALSE, "Is Write?"=FALSE, "Inactive Parent?"=FALSE, "Unwired?"=FALSE}, {"Label"="Fixed-Point Representation", "Tag"="Fixed-Point Representation", "Property Type"=enum."Private", "Indent"=0, "Can Read?"=FALSE, "Can Write?"=FALSE, "Is Read?"=FALSE, "Is Write?"=FALSE, "Inactive Parent?"=TRUE, "Unwired?"=FALSE}, {"Label"="Include Overflow Status?", "Tag"="633b01f.Fixed-Point Representation:Include Overflow Status?", "Property Type"=enum."Private", "Indent"=1, "Can Read?"=TRUE, "Can Write?"=TRUE, "Is Read?"=FALSE, "Is Write?"=FALSE, "Inactive Parent?"=FALSE, "Unwired?"=FALSE}, {"Label"="Increment Key Binding", "Tag"="633b010.Increment Key Binding", "Property Type"=enum."Base", "Indent"=0, "Can Read?"=TRUE, "Can Write?"=TRUE, "Is Read?"=FALSE, "Is Write?"=FALSE, "Inactive Parent?"=FALSE, "Unwired?"=FALSE}, {"Label"="Representation", "Tag"="633b003.Representation", "Property Type"=enum."Scripting", "Indent"=0, "Can Read?"=TRUE, "Can Write?"=TRUE, "Is Read?"=FALSE, "Is Write?"=FALSE, "Inactive Parent?"=FALSE, "Unwired?"=FALSE}, {"Label"="Response to Value Outside Limits", "Tag"="633b00b.Response to Value Outside Limits", "Property Type"=enum."Base", "Indent"=0, "Can Read?"=TRUE, "Can Write?"=TRUE, "Is Read?"=FALSE, "Is Write?"=FALSE, "Inactive Parent?"=FALSE, "Unwired?"=FALSE}, {"Label"="Increment", "Tag"="633b00e.Response to Value Outside Limits:Increment", "Property Type"=enum."Base", "Indent"=1, "Can Read?"=TRUE, "Can Write?"=TRUE, "Is Read?"=FALSE, "Is Write?"=FALSE, "Inactive Parent?"=FALSE, "Unwired?"=FALSE}, {"Label"="Maximum", "Tag"="633b00c.Response to Value Outside Limits:Maximum", "Property Type"=enum."Base", "Indent"=1, "Can Read?"=TRUE, "Can Write?"=TRUE, "Is Read?"=FALSE, "Is Write?"=FALSE, "Inactive Parent?"=FALSE, "Unwired?"=FALSE}, {"Label"="Minimum", "Tag"="633b00d.Response to Value Outside Limits:Minimum", "Property Type"=enum."Base", "Indent"=1, "Can Read?"=TRUE, "Can Write?"=TRUE, "Is Read?"=FALSE, "Is Write?"=FALSE, "Inactive Parent?"=FALSE, "Unwired?"=FALSE}, {"Label"="Unit Label", "Tag"="633b00a.Unit Label", "Property Type"=enum."Base", "Indent"=0, "Can Read?"=TRUE, "Can Write?"=FALSE, "Is Read?"=FALSE, "Is Write?"=FALSE, "Inactive Parent?"=FALSE, "Unwired?"=FALSE}, {"Label"="Display Format", "Tag"="633bc06.Display Format", "Property Type"=enum."Base", "Indent"=0, "Can Read?"=TRUE, "Can Write?"=TRUE, "Is Read?"=FALSE, "Is Write?"=FALSE, "Inactive Parent?"=FALSE, "Unwired?"=FALSE}, {"Label"="Format", "Tag"="633bc07.Display Format:Format", "Property Type"=enum."Base", "Indent"=1, "Can Read?"=TRUE, "Can Write?"=TRUE, "Is Read?"=FALSE, "Is Write?"=FALSE, "Inactive Parent?"=FALSE, "Unwired?"=FALSE}, {"Label"="Precision", "Tag"="633bc08.Display Format:Precision", "Property Type"=enum."Base", "Indent"=1, "Can Read?"=TRUE, "Can Write?"=TRUE, "Is Read?"=FALSE, "Is Write?"=FALSE, "Inactive Parent?"=FALSE, "Unwired?"=FALSE}, {"Label"="Format String", "Tag"="633bc05.Format String", "Property Type"=enum."Base", "Indent"=0, "Can Read?"=TRUE, "Can Write?"=TRUE, "Is Read?"=FALSE, "Is Write?"=FALSE, "Inactive Parent?"=FALSE, "Unwired?"=FALSE}, {"Label"="Hide Text", "Tag"="633bc09.Hide Text", "Property Type"=enum."Private", "Indent"=0, "Can Read?"=TRUE, "Can Write?"=TRUE, "Is Read?"=FALSE, "Is Write?"=FALSE, "Inactive Parent?"=FALSE, "Unwired?"=FALSE}, {"Label"="Increment/Decrement Visible?", "Tag"="633bc04.Increment/Decrement Visible?", "Property Type"=enum."Base", "Indent"=0, "Can Read?"=TRUE, "Can Write?"=TRUE, "Is Read?"=FALSE, "Is Write?"=FALSE, "Inactive Parent?"=FALSE, "Unwired?"=FALSE}, {"Label"="Numeric Text", "Tag"="633bc03.Numeric Text", "Property Type"=enum."Base", "Indent"=0, "Can Read?"=TRUE, "Can Write?"=FALSE, "Is Read?"=FALSE, "Is Write?"=FALSE, "Inactive Parent?"=FALSE, "Unwired?"=FALSE}, {"Label"="Radix Visible?", "Tag"="633bc02.Radix Visible?", "Property Type"=enum."Base", "Indent"=0, "Can Read?"=TRUE, "Can Write?"=TRUE, "Is Read?"=FALSE, "Is Write?"=FALSE, "Inactive Parent?"=FALSE, "Unwired?"=FALSE}, {"Label"="Text Width", "Tag"="633bc01.Text Width", "Property Type"=enum."Base", "Indent"=0, "Can Read?"=TRUE, "Can Write?"=TRUE, "Is Read?"=FALSE, "Is Write?"=FALSE, "Inactive Parent?"=FALSE, "Unwired?"=FALSE}] ("Properties for Tree Out"), s=w59, f=w51) -> (s? t:f=w57:T5)
      n21 = call <userlib>:"Current VIs Reference__ogtk.vi"() -> ("Current VI's reference"=w53:refnum<vi>)  [unwired: 5 in]
      n22 = call "Property Tree_Populate Trees.vi"("Close Items"=w50, "VI Ref"=w53, "Filter"="", "Action"=w56, "Error In"=w45, "Tree Refs"=w55, "Show"=w54, "Properties for Tree In"=w57) -> ("error out"=w48:errorcluster)  [unwired: 3 in]
      n23 = call "Tree_Setup for dialog.vi"("Action"=w56, "error in"=w48, "Tree Ref"=w55) -> ("error out"=w46:errorcluster)  [unwired: 7 in, 1 out]
      n24 = call "Dialog Window Setup.vi"("Action"=enum16{"Pre-Populate", "Post-Populate"}."Post-Populate", "error in"=w46, "Dialog VI Ref In [Parent]"=w49) -> ("error out"=w43:errorcluster)  [unwired: 7 in, 1 out]
      n25 = control-ref of="Filter"() -> (w44:refnum<vi>)
      n26 = call "Dialog_Setup Filter String.vi"("Action"=w41, "error in"=w43, "Filter String Ref"=w44) -> ("error out"=w42:errorcluster)  [unwired: 7 in, 1 out]
    }
  }
  n27 = call <vilib>:"Simple Error Handler.vi"("error in (no error)"=w2) -> ()  [unwired: 4 in, 5 out]
  n28 = while {
    tunnel: w13 -> [w65]
    tunnel: [w64] -> w20
    tunnel: [w63] -> w16
    tunnel: w18 -> [w63]
    tunnel: w9 -> [w62]
    shift-right: [w60] -> _
    shift-left: w6 -> [w61]
    stop <- w66 stop-if-true
    n29 = event shown="[1] \"Property Display\", \"Filter\": Value Change" {
      selector: _ -> [_ _ _ _ _ _ _ _]
      dyn-events: _ -> [_ _ _ _ _ _ _ _]
      timeout: _ -> [_ _ _ _ _ _ _ _]
      tunnel: [w71 _ _ _ _ _ w132 w138] -> w66
      tunnel: w65 -> [w68 w76 w86 w106 w110 _ _ _]
      tunnel: [TRUE _ _ _ _ _ FALSE _] -> w64
      tunnel: w62 -> [w67 w84 _ _ _ _ _ _]
      tunnel: w61 -> [w69 w77 w87 w104 w112 w126 w131 w136]
      tunnel: [w69 w75 w87 w104 w112 w126 w131 w136] -> w60
      event Value Change {
        n30 = event-data() -> ("NewVal"=w71:T2)  [unwired: 1 in]
        n31 = call "Property Tree_Select on Enter.vi"("Save Action"=w67, "Tree Ref"=w68) -> ()  [unwired: 10 in]
      }
      event "Property Display", "Filter": Value Change {
        w72 = FALSE  # Close Items
        n32 = event-data() -> ()  [unwired: 1 in, 1 out]
        n33 = call "Properties_Update RW From Value.vi"("Properties for Tree In"=w77) -> ("Properties for Tree Out"=w75:T5)  [unwired: 10 in]
        n34 = Equal?(x="Filter..." ("Default Value"), y="Filter") -> (x = y?=w83:bool)
        n35 = Select(t="", s=w83, f="Filter") -> (s? t:f=w79:string)
        n36 = call <userlib>:"Current VIs Reference__ogtk.vi"() -> ("Current VI's reference"=w78:refnum<vi>)  [unwired: 5 in]
        n37 = call "Property Tree_Populate Trees.vi"("Close Items"=w72, "VI Ref"=w78, "Filter"=w79, "Action"=w84, "Tree Refs"=w76, "Show"="Property Display", "Properties for Tree In"=w75) -> ()  [unwired: 4 in, 1 out]
        n38 = call "INI_Dialog display options.vi"("File Action"=enum16{"Read", "Write"}."Write", "Display Options"="Property Display") -> ()  [unwired: 9 in, 1 out]
      }
      event "Filter": Key Down? {
        n39 = event-data() -> ("ScanCode"=w89:i16)  [unwired: 1 in]
        n40 = control-ref of="Done"() -> (w85:refnum<vi>)
        n41 = Index Array(array=w86) -> (element=w88:refnum<vi>)  [unwired: 1 in]
        n42 = case shown="Default" w89 {
          tunnel: [_ TRUE TRUE] -> w90
          tunnel: w88 -> [_ w96 w102]
          tunnel: w86 -> [_ w93 w99]
          tunnel: w85 -> [_ w91 w97]
          frame Default {
          }
          frame 15, 80 {
            # "on down arrow [80] or tab [15], put key focus on tree control and select first item"
            # "Down Arrow, Tab"
            n43 = call "Tree_Select first or last item.vi"("Select Item"=enum16{"First", "Last"}."First", "Done Ref"=w91, "Tree Ref"=w96) -> ("Tree Ref Out"=w92:refnum<vi>)  [unwired: 7 in, 1 out]
            n44 = call "Tree Sync_Sync Top Item.vi"("Changed Tree Control Ref"=w92, "All Tree Control Refs"=w93) -> ()  [unwired: 9 in, 1 out]
          }
          frame 72 {
            # "Up Arrow"
            n45 = call "Tree_Select first or last item.vi"("Select Item"=enum16{"First", "Last"}."Last", "Done Ref"=w97, "Tree Ref"=w102) -> ("Tree Ref Out"=w98:refnum<vi>)  [unwired: 7 in, 1 out]
            n46 = call "Tree Sync_Sync Top Item.vi"("Changed Tree Control Ref"=w98, "All Tree Control Refs"=w99) -> ()  [unwired: 9 in, 1 out]
          }
        }
        n47 = event-data("Discard?"=w90) -> ()  [unwired: 1 in, 1 out]
      }
      event "Boolean": Value Change {
        n48 = event-data() -> ()  [unwired: 1 in, 1 out]
        n49 = Index Array(array=w106) -> (element=w105:refnum<vi>)  [unwired: 1 in]
        n50 = call "Property Dialog_Select Unwired Terminals.vi"("Select Unwired"="Boolean", "Properties for Tree In"=w104, "Tree Ref"=w105) -> ()  [unwired: 9 in]
      }
      event "Main Tree": Key Down? {
        n51 = event-data() -> ("VKey"=w111:T7, "ScanCode"=w108:i16)  [unwired: 1 in]
        n52 = Index Array(array=w110) -> (element=w109:refnum<vi>)  [unwired: 1 in]
        n53 = case shown="\"Up\"" w111 {
          tunnel: [_ w113 w118 w121] -> w107
          tunnel: w109 -> [_ _ w119 w122]
          tunnel: w108 -> [_ w114 _ _]
          frame Default {
          }
          frame "ASCII" {
            n54 = case shown="15" w114 {
              tunnel: [_ TRUE ("Discard?")] -> w113
              frame 0, Default {
              }
              frame 15 {
                # "to tab off tree control required this"
                # "TAB"
                n55 = control-ref of="Done"() -> (w116:refnum<vi>)
                n56 = property class="Bool"(reference=w116, "Key Focus"=TRUE) -> ()  [unwired: 1 in, 2 out]
              }
            }
          }
          frame "Up" {
            # "#TODO listbox key navigation includes divider, which is confusing. Handle this better"
            n57 = call "Tree_Go to next displayed item.vi"("Direction"=enum16{"Down", "Up"}."Up", "Tree ref"=w119) -> ("discard"=w118:bool)  [unwired: 7 in, 2 out]
          }
          frame "Down" {
            n58 = call "Tree_Go to next displayed item.vi"("Direction"=enum16{"Down", "Up"}."Down", "Tree ref"=w122) -> ("discard"=w121:bool)  [unwired: 7 in, 2 out]
          }
        }
        n59 = event-data("Discard?"=w107) -> ()  [unwired: 1 in, 1 out]
      }
      event Key Down? {
        # "Force tab loop filter-tree-done-filter"
        n60 = event-data() -> ("ScanCode"=w124:i16)  [unwired: 1 in]
        n61 = case shown="15" w124 {
          tunnel: [_ TRUE ("Discard?")] -> w125
          frame 0, Default {
          }
          frame 15 {
            n62 = control-ref of="Filter"() -> (w127:refnum<vi>)
            n63 = property class="Str"(reference=w127, "Key Focus"=TRUE) -> ()  [unwired: 1 in, 2 out]
          }
        }
        n64 = event-data("Discard?"=w125) -> ()  [unwired: 1 in, 1 out]
      }
      event Key Down? {
        # "Quit on escape"
        n65 = event-data() -> ("VKey"=w133:T7)  [unwired: 1 in]
        n66 = case shown="Default" w133 {
          tunnel: [FALSE TRUE] -> w132
          frame Default {
          }
          frame "Escape" {
            # "Close window and return no value on esc"
          }
        }
        n67 = event-data("Discard?"=w132) -> ()  [unwired: 1 in, 1 out]
      }
      event Panel Close? {
        w138 = TRUE
        # "close and return no value on panel close"
        n68 = event-data() -> ()  [unwired: 1 in, 1 out]
        n69 = call "Is VI Running Top Level.vi"() -> ("Top Level?"=w137:bool)  [unwired: 5 in]
        n70 = case shown="False" w137 {
          frame False {
            n71 = invoke class="VI" method="FP.Close"() -> ()  [unwired: 3 in, 3 out]
          }
          frame True {
          }
        }
        n72 = event-data("Discard?"=w138) -> ()  [unwired: 1 in, 1 out]
      }
    }
  }
  n73 = call "Is VI Running Top Level.vi"() -> ("Top Level?"=w14:bool)  [unwired: 5 in]
  n74 = case shown="True" w20 {
    tunnel: w9 -> [_ w143]
    tunnel: w13 -> [_ w142]
    tunnel: [_ "Placement"] -> w17
    tunnel: [T3 [] ("Property Array Out") w140] -> w8
    frame False {
    }
    frame True {
      n75 = case shown="\"Properties Rearrange\"" w143 {
        tunnel: w142 -> [_ w146 _]
        tunnel: [w145 w147 w149] -> w140
        frame "Properties Remove" {
          n76 = call "Property Tree_Value Engine.vi"("Save Action"=T8."Read" ("Action")) -> ("Property Array Out"=w145:T3)  [unwired: 8 in, 2 out]
        }
        frame "Properties Rearrange" {
          n77 = call "Properties for Rearrange.vi"("Tree Controls"=w146) -> ("Property Array Out"=w147:T3)  [unwired: 9 in, 1 out]
        }
        frame Default {
          n78 = call "Property Tree_Value Engine.vi"("Save Action"=T8."Read" ("Action")) -> ("Property Array Out"=w149:T3)  [unwired: 8 in, 2 out]
        }
      }
    }
  }
  "Placement Out" <- w17
  n79 = case shown="False" w14 {
    tunnel: w16 -> [w151 w152]
    tunnel: [w150 w152] -> w15
    frame False {
      n80 = invoke class="VI" method="FP.Close"(reference=w151) -> (reference out=w150:refnum<vi>)  [unwired: 2 in, 2 out]
    }
    frame True {
    }
  }
  n81 = call "FP splitter mode handler.vi"("Mode"=enum16{"Run", "Development"}."Development", "VI Ref In"=w15) -> ()  [unwired: 8 in, 2 out]
  n82 = call "Order Properties from Dialog.vi"("Original Properties"=w6, "Property Array In"=w8) -> ("Property Array Out"=→"Property Array Out":T3)  [unwired: 9 in]
  "Error Out" <- "Error In"
